vi "函数类型3测试.vi"() -> ()   [LabVIEW 2010]
uses:
  全局量/试验配置信息.vi
panel:
  out "合格？":bool[](array[boolean])
  in  "第几组数据":i32
  out "D_IN_1 2":string[][](table) caption="表格"
  in  "加载文件名称":string
  out "配置文件路径":path
  out "配置文件目录 2":path
  out "配置文件目录":path
  in  "加载配置文件":u16(ring)
  in  "同步_A2":i32
  in  "同步_A1":i32
  in  "数组_输入值":enum16{"0", "1"}[](array[ring])
  in  "数组_选择?":bool[](array[boolean])
  in  "btn_置1_5":bool
  in  "btn_置1_4":bool
  in  "btn_置1_3":bool
  in  "btn_置1_2":bool
  in  "btn_全选_5":bool
  in  "btn_全选_4":bool
  in  "btn_全选_3":bool
  in  "btn_全选_2":bool
  in  "btn_置1_1":bool
  in  "btn_全选_1":bool
  in  "CAN端口":u16
  out "light_80":bool
  out "light_79":bool
  out "light_78":bool
  out "light_77":bool
  out "light_76":bool
  out "light_75":bool
  out "light_74":bool
  out "light_73":bool
  out "light_72":bool
  out "light_71":bool
  out "light_70":bool
  out "light_69":bool
  out "light_68":bool
  out "light_67":bool
  out "light_66":bool
  out "light_65":bool
  in  "输入值_73":enum16{"0", "1"}(ring)
  in  "输入值_80":enum16{"0", "1"}(ring)
  in  "输入值_79":enum16{"0", "1"}(ring)
  in  "输入值_78":enum16{"0", "1"}(ring)
  in  "输入值_77":enum16{"0", "1"}(ring)
  in  "输入值_76":enum16{"0", "1"}(ring)
  in  "输入值_75":enum16{"0", "1"}(ring)
  in  "输入值_74":enum16{"0", "1"}(ring)
  in  "输入值_65":enum16{"0", "1"}(ring)
  in  "输入值_72":enum16{"0", "1"}(ring)
  in  "输入值_71":enum16{"0", "1"}(ring)
  in  "输入值_70":enum16{"0", "1"}(ring)
  in  "输入值_69":enum16{"0", "1"}(ring)
  in  "输入值_68":enum16{"0", "1"}(ring)
  in  "输入值_67":enum16{"0", "1"}(ring)
  in  "输入值_66":enum16{"0", "1"}(ring)
  in  "单选_第73路":bool
  in  "单选_第80路":bool
  in  "单选_第79路":bool
  in  "单选_第78路":bool
  in  "单选_第77路":bool
  in  "单选_第76路":bool
  in  "单选_第75路":bool
  in  "单选_第74路":bool
  in  "单选_第65路":bool
  in  "单选_第72路":bool
  in  "单选_第71路":bool
  in  "单选_第70路":bool
  in  "单选_第69路":bool
  in  "单选_第68路":bool
  in  "单选_第67路":bool
  in  "单选_第66路":bool
  out "light_64":bool
  out "light_63":bool
  out "light_62":bool
  out "light_61":bool
  out "light_60":bool
  out "light_59":bool
  out "light_58":bool
  out "light_57":bool
  out "light_56":bool
  out "light_55":bool
  out "light_54":bool
  out "light_53":bool
  out "light_52":bool
  out "light_51":bool
  out "light_50":bool
  out "light_49":bool
  in  "输入值_57":enum16{"0", "1"}(ring)
  in  "输入值_64":enum16{"0", "1"}(ring)
  in  "输入值_63":enum16{"0", "1"}(ring)
  in  "输入值_62":enum16{"0", "1"}(ring)
  in  "输入值_61":enum16{"0", "1"}(ring)
  in  "输入值_60":enum16{"0", "1"}(ring)
  in  "输入值_59":enum16{"0", "1"}(ring)
  in  "输入值_58":enum16{"0", "1"}(ring)
  in  "输入值_49":enum16{"0", "1"}(ring)
  in  "输入值_56":enum16{"0", "1"}(ring)
  in  "输入值_55":enum16{"0", "1"}(ring)
  in  "输入值_54":enum16{"0", "1"}(ring)
  in  "输入值_53":enum16{"0", "1"}(ring)
  in  "输入值_52":enum16{"0", "1"}(ring)
  in  "输入值_51":enum16{"0", "1"}(ring)
  in  "输入值_50":enum16{"0", "1"}(ring)
  in  "单选_第57路":bool
  in  "单选_第64路":bool
  in  "单选_第63路":bool
  in  "单选_第62路":bool
  in  "单选_第61路":bool
  in  "单选_第60路":bool
  in  "单选_第59路":bool
  in  "单选_第58路":bool
  in  "单选_第49路":bool
  in  "单选_第56路":bool
  in  "单选_第55路":bool
  in  "单选_第54路":bool
  in  "单选_第53路":bool
  in  "单选_第52路":bool
  in  "单选_第51路":bool
  in  "单选_第50路":bool
  out "light_48":bool
  out "light_47":bool
  out "light_46":bool
  out "light_45":bool
  out "light_44":bool
  out "light_43":bool
  out "light_42":bool
  out "light_41":bool
  out "light_40":bool
  out "light_39":bool
  out "light_38":bool
  out "light_37":bool
  out "light_36":bool
  out "light_35":bool
  out "light_34":bool
  out "light_33":bool
  in  "输入值_41":enum16{"0", "1"}(ring)
  in  "输入值_48":enum16{"0", "1"}(ring)
  in  "输入值_47":enum16{"0", "1"}(ring)
  in  "输入值_46":enum16{"0", "1"}(ring)
  in  "输入值_45":enum16{"0", "1"}(ring)
  in  "输入值_44":enum16{"0", "1"}(ring)
  in  "输入值_43":enum16{"0", "1"}(ring)
  in  "输入值_42":enum16{"0", "1"}(ring)
  in  "输入值_33":enum16{"0", "1"}(ring)
  in  "输入值_40":enum16{"0", "1"}(ring)
  in  "输入值_39":enum16{"0", "1"}(ring)
  in  "输入值_38":enum16{"0", "1"}(ring)
  in  "输入值_37":enum16{"0", "1"}(ring)
  in  "输入值_36":enum16{"0", "1"}(ring)
  in  "输入值_35":enum16{"0", "1"}(ring)
  in  "输入值_34":enum16{"0", "1"}(ring)
  in  "单选_第41路":bool
  in  "单选_第48路":bool
  in  "单选_第47路":bool
  in  "单选_第46路":bool
  in  "单选_第45路":bool
  in  "单选_第44路":bool
  in  "单选_第43路":bool
  in  "单选_第42路":bool
  in  "单选_第33路":bool
  in  "单选_第40路":bool
  in  "单选_第39路":bool
  in  "单选_第38路":bool
  in  "单选_第37路":bool
  in  "单选_第36路":bool
  in  "单选_第35路":bool
  in  "单选_第34路":bool
  out "light_32":bool
  out "light_31":bool
  out "light_30":bool
  out "light_29":bool
  out "light_28":bool
  out "light_27":bool
  out "light_26":bool
  out "light_25":bool
  out "light_24":bool
  out "light_23":bool
  out "light_22":bool
  out "light_21":bool
  out "light_20":bool
  out "light_19":bool
  out "light_18":bool
  out "light_17":bool
  in  "输入值_25":enum16{"0", "1"}(ring)
  in  "输入值_32":enum16{"0", "1"}(ring)
  in  "输入值_31":enum16{"0", "1"}(ring)
  in  "输入值_30":enum16{"0", "1"}(ring)
  in  "输入值_29":enum16{"0", "1"}(ring)
  in  "输入值_28":enum16{"0", "1"}(ring)
  in  "输入值_27":enum16{"0", "1"}(ring)
  in  "输入值_26":enum16{"0", "1"}(ring)
  in  "输入值_17":enum16{"0", "1"}(ring)
  in  "输入值_24":enum16{"0", "1"}(ring)
  in  "输入值_23":enum16{"0", "1"}(ring)
  in  "输入值_22":enum16{"0", "1"}(ring)
  in  "输入值_21":enum16{"0", "1"}(ring)
  in  "输入值_20":enum16{"0", "1"}(ring)
  in  "输入值_19":enum16{"0", "1"}(ring)
  in  "输入值_18":enum16{"0", "1"}(ring)
  in  "单选_第25路":bool
  in  "单选_第32路":bool
  in  "单选_第31路":bool
  in  "单选_第30路":bool
  in  "单选_第29路":bool
  in  "单选_第28路":bool
  in  "单选_第27路":bool
  in  "单选_第26路":bool
  in  "单选_第17路":bool
  in  "单选_第24路":bool
  in  "单选_第23路":bool
  in  "单选_第22路":bool
  in  "单选_第21路":bool
  in  "单选_第20路":bool
  in  "单选_第19路":bool
  in  "单选_第18路":bool
  in  "D_IN_5":string[][](table) caption="表格"
  in  "D_IN_4":string[][](table) caption="表格"
  in  "D_IN_3":string[][](table) caption="表格"
  in  "D_IN_2":string[][](table) caption="表格"
  out "light_16":bool
  out "light_15":bool
  out "light_14":bool
  out "light_13":bool
  out "light_12":bool
  out "light_11":bool
  out "light_10":bool
  out "light_9":bool
  out "light_8":bool
  out "light_7":bool
  out "light_6":bool
  out "light_5":bool
  out "light_4":bool
  out "light_3":bool
  out "light_2":bool
  out "light_1":bool
  in  "输入值_9":enum16{"0", "1"}(ring)
  in  "输入值_16":enum16{"0", "1"}(ring)
  in  "输入值_15":enum16{"0", "1"}(ring)
  in  "输入值_14":enum16{"0", "1"}(ring)
  in  "输入值_13":enum16{"0", "1"}(ring)
  in  "输入值_12":enum16{"0", "1"}(ring)
  in  "输入值_11":enum16{"0", "1"}(ring)
  in  "输入值_10":enum16{"0", "1"}(ring)
  in  "输入值_1":enum16{"0", "1"}(ring)
  in  "输入值_8":enum16{"0", "1"}(ring)
  in  "输入值_7":enum16{"0", "1"}(ring)
  in  "输入值_6":enum16{"0", "1"}(ring)
  in  "输入值_5":enum16{"0", "1"}(ring)
  in  "输入值_4":enum16{"0", "1"}(ring)
  in  "输入值_3":enum16{"0", "1"}(ring)
  in  "输入值_2":enum16{"0", "1"}(ring)
  in  "单选_第9路":bool
  in  "单选_第16路":bool
  in  "单选_第15路":bool
  in  "单选_第14路":bool
  in  "单选_第13路":bool
  in  "单选_第12路":bool
  in  "单选_第11路":bool
  in  "单选_第10路":bool
  in  "单选_第1路":bool
  in  "单选_第8路":bool
  in  "单选_第7路":bool
  in  "单选_第6路":bool
  in  "单选_第5路":bool
  in  "单选_第4路":bool
  in  "单选_第3路":bool
  in  "单选_第2路":bool
  in  "D_IN_1":string[][](table) caption="表格"
  out "关闭？":bool
  out "测试结论":string
  in  "btn_置0":bool
  in  "btn_置1":bool
  in  "btn_反选":bool
  in  "btn_全选":bool
  in  "btn_关闭":bool
  in  "btn_开始试验":bool
  # "第一组数字量测试"
  # "第二组数字量测试"
  # "第三组数字量测试"
  # "第四组数字量测试"
  # "第五组数字量测试"
  # "加载配置文件："
  # "测试结论："
  # "80"
  # "80"
  # "80"
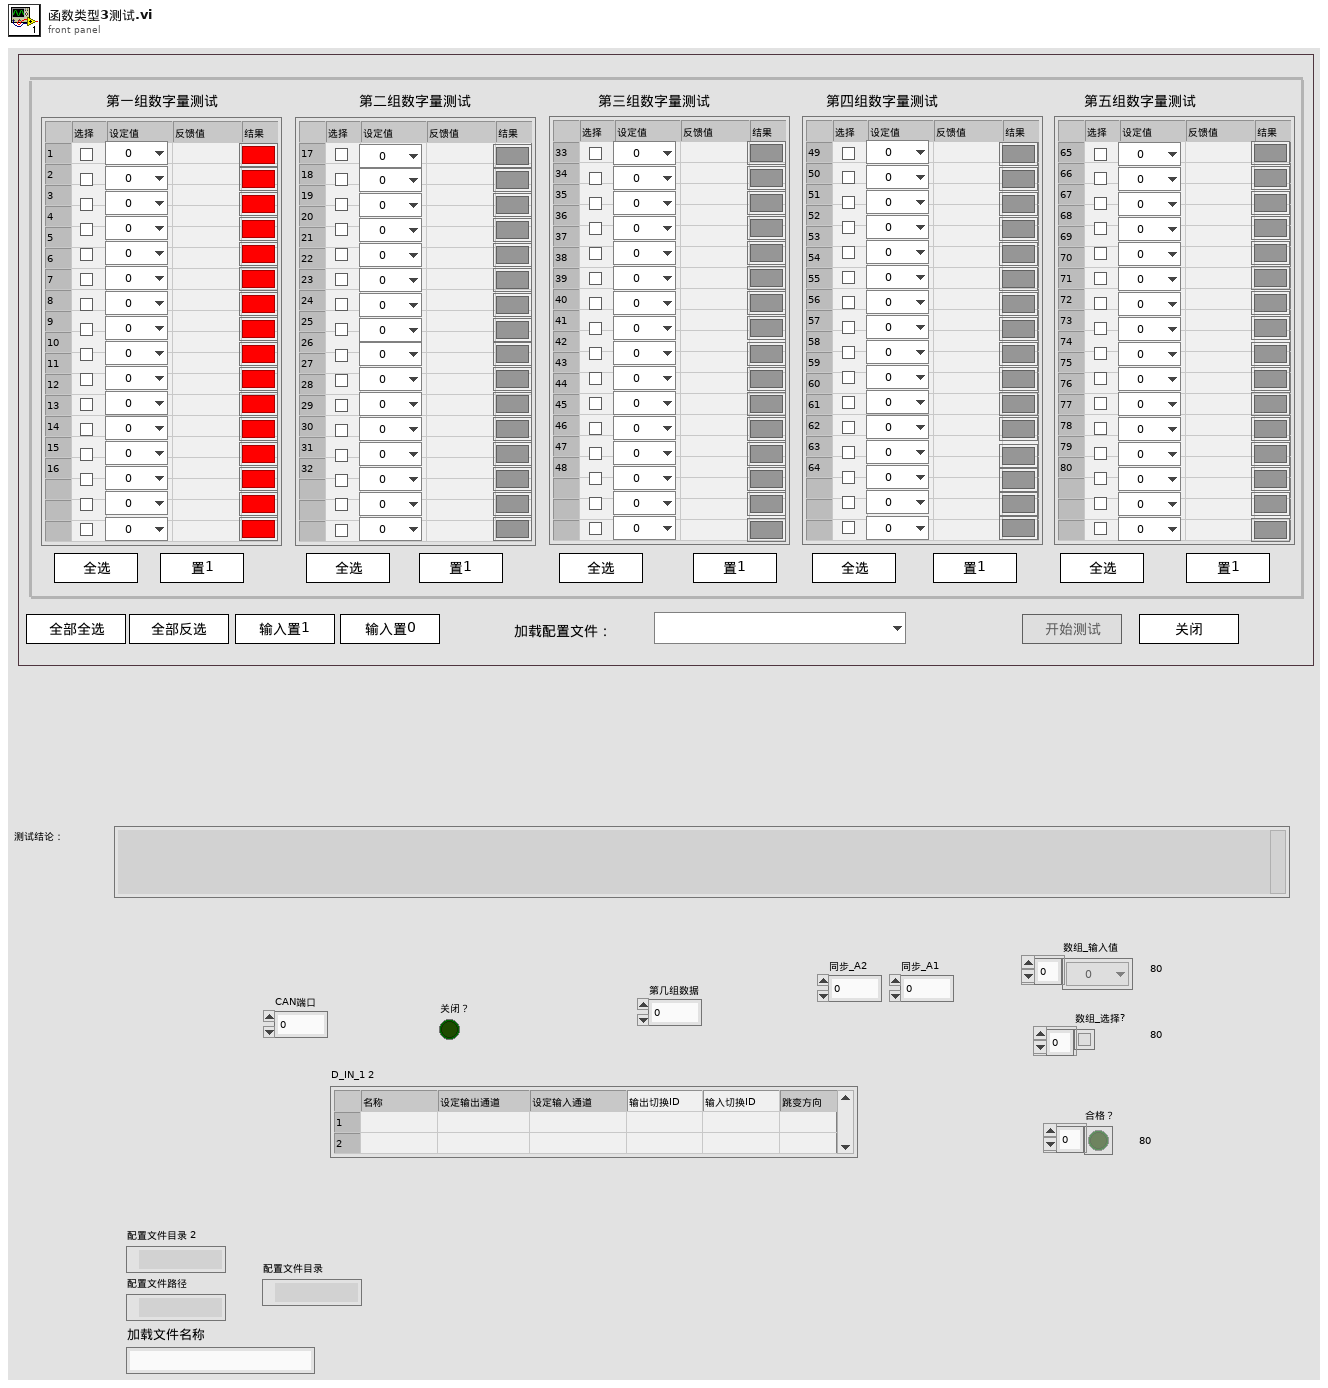
[diagram p1: front panel]
types:
  T1 = enum8{"Enabled", "Disabled", "Disabled and Grayed Out"}
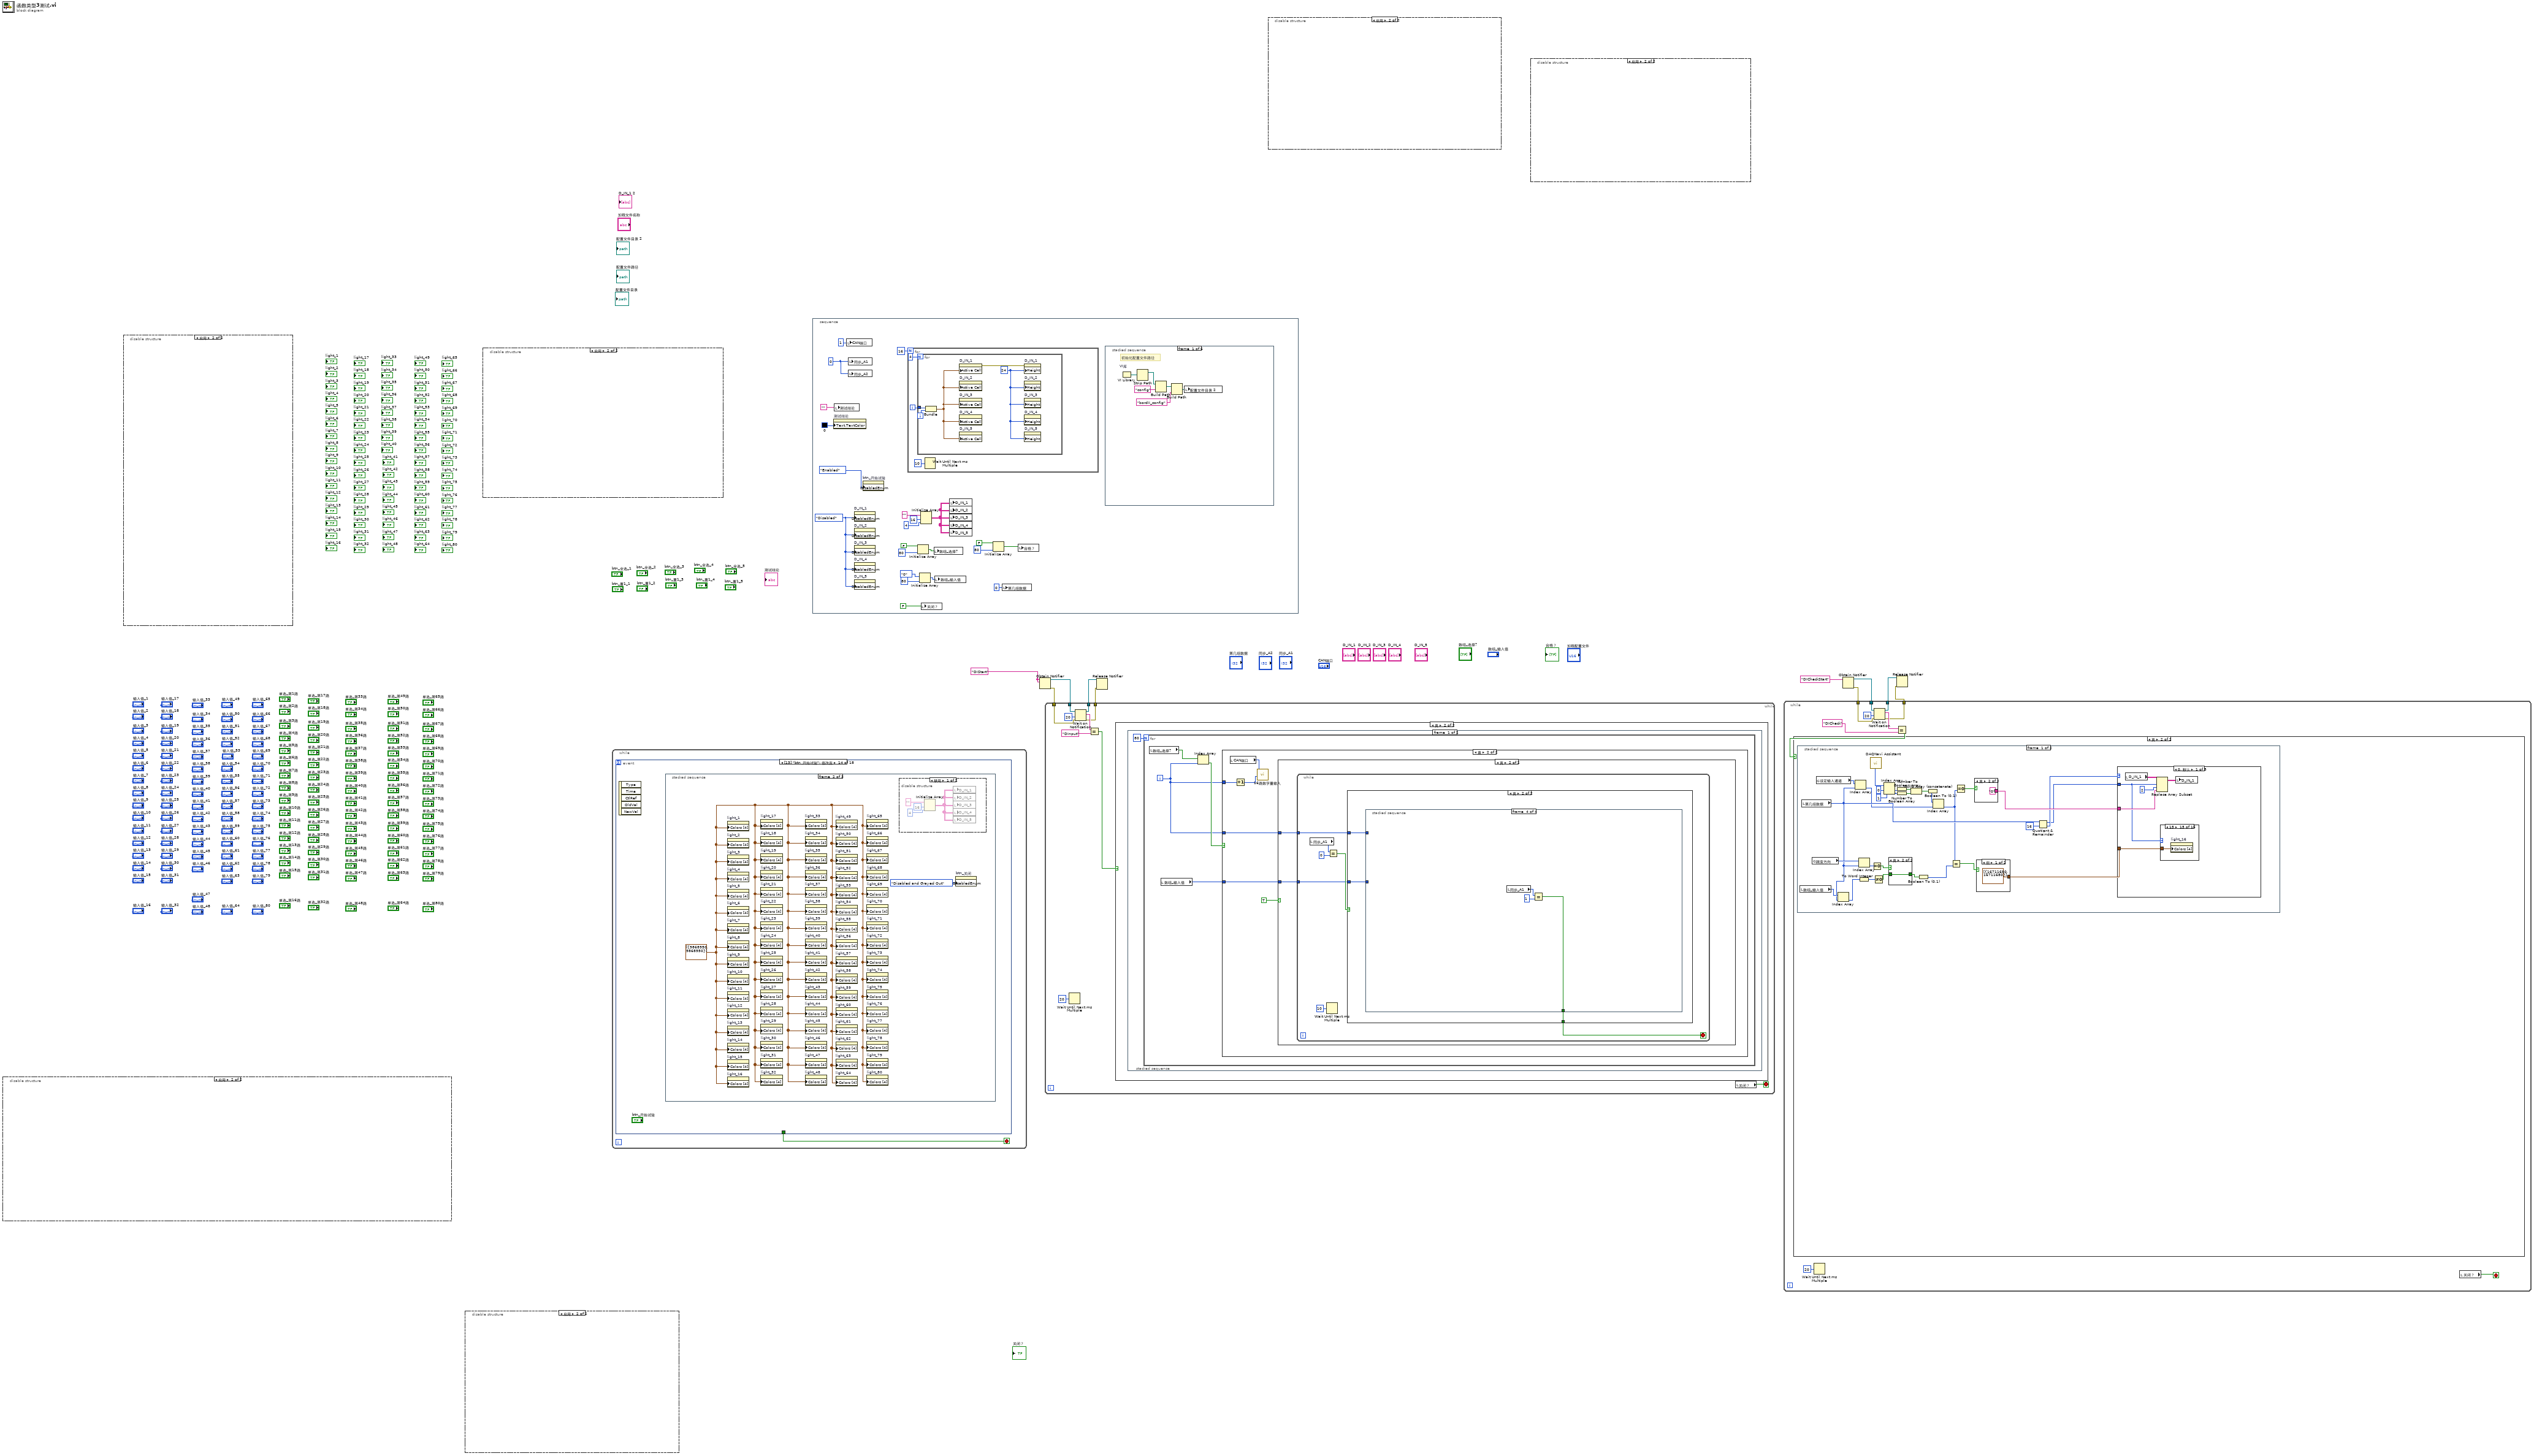
[diagram p0: block diagram]
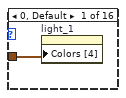
[diagram p3: hidden frame]
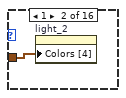
[diagram p4: hidden frame]
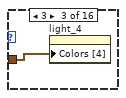
[diagram p5: hidden frame]
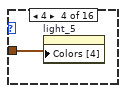
[diagram p6: hidden frame]
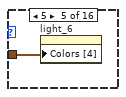
[diagram p7: hidden frame]
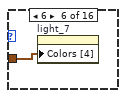
[diagram p8: hidden frame]
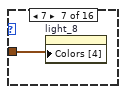
[diagram p9: hidden frame]
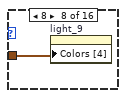
[diagram p10: hidden frame]
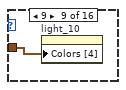
[diagram p11: hidden frame]
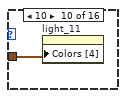
[diagram p12: hidden frame]
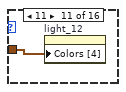
[diagram p13: hidden frame]
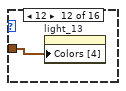
[diagram p14: hidden frame]
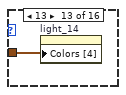
[diagram p15: hidden frame]
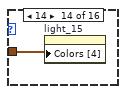
[diagram p16: hidden frame]
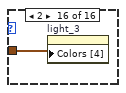
[diagram p17: hidden frame]
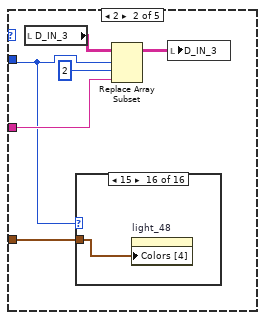
[diagram p18: hidden frame]
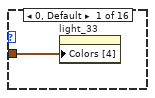
[diagram p19: hidden frame]
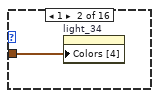
[diagram p20: hidden frame]
diagram:
  w1 = "DICheckStart" ("名称（未命名）")
  w2 = "DIStart" ("名称（未命名）")
  n1 = disable-structure shown="启用" {
    frame Disabled {
      n2 = local read "单选_第1路"() -> ()  [unwired: 1 in]
      n3 = local read "单选_第2路"() -> ()  [unwired: 1 in]
      n4 = local read "单选_第3路"() -> ()  [unwired: 1 in]
      n5 = local read "单选_第4路"() -> ()  [unwired: 1 in]
      n6 = local read "单选_第5路"() -> ()  [unwired: 1 in]
      n7 = local read "单选_第6路"() -> ()  [unwired: 1 in]
      n8 = local read "单选_第7路"() -> ()  [unwired: 1 in]
      n9 = local read "单选_第8路"() -> ()  [unwired: 1 in]
      n10 = local read "单选_第9路"() -> ()  [unwired: 1 in]
      n11 = local read "单选_第10路"() -> ()  [unwired: 1 in]
      n12 = local read "单选_第11路"() -> ()  [unwired: 1 in]
      n13 = local read "单选_第12路"() -> ()  [unwired: 1 in]
      n14 = local read "单选_第13路"() -> ()  [unwired: 1 in]
      n15 = local read "单选_第14路"() -> ()  [unwired: 1 in]
      n16 = local read "单选_第15路"() -> ()  [unwired: 1 in]
      n17 = local read "单选_第16路"() -> ()  [unwired: 1 in]
      n18 = local read "单选_第17路"() -> ()  [unwired: 1 in]
      n19 = local read "单选_第18路"() -> ()  [unwired: 1 in]
      n20 = local read "单选_第19路"() -> ()  [unwired: 1 in]
      n21 = local read "单选_第20路"() -> ()  [unwired: 1 in]
      n22 = local read "单选_第21路"() -> ()  [unwired: 1 in]
      n23 = local read "单选_第22路"() -> ()  [unwired: 1 in]
      n24 = local read "单选_第23路"() -> ()  [unwired: 1 in]
      n25 = local read "单选_第24路"() -> ()  [unwired: 1 in]
      n26 = local read "单选_第25路"() -> ()  [unwired: 1 in]
      n27 = local read "单选_第26路"() -> ()  [unwired: 1 in]
      n28 = local read "单选_第27路"() -> ()  [unwired: 1 in]
      n29 = local read "单选_第28路"() -> ()  [unwired: 1 in]
      n30 = local read "单选_第29路"() -> ()  [unwired: 1 in]
      n31 = local read "单选_第30路"() -> ()  [unwired: 1 in]
      n32 = local read "单选_第31路"() -> ()  [unwired: 1 in]
      n33 = local read "单选_第32路"() -> ()  [unwired: 1 in]
      n34 = local read "单选_第33路"() -> ()  [unwired: 1 in]
      n35 = local read "单选_第34路"() -> ()  [unwired: 1 in]
      n36 = local read "单选_第35路"() -> ()  [unwired: 1 in]
      n37 = local read "单选_第36路"() -> ()  [unwired: 1 in]
      n38 = local read "单选_第37路"() -> ()  [unwired: 1 in]
      n39 = local read "单选_第38路"() -> ()  [unwired: 1 in]
      n40 = local read "单选_第39路"() -> ()  [unwired: 1 in]
      n41 = local read "单选_第40路"() -> ()  [unwired: 1 in]
      n42 = local read "单选_第41路"() -> ()  [unwired: 1 in]
      n43 = local read "单选_第42路"() -> ()  [unwired: 1 in]
      n44 = local read "单选_第43路"() -> ()  [unwired: 1 in]
      n45 = local read "单选_第44路"() -> ()  [unwired: 1 in]
      n46 = local read "单选_第45路"() -> ()  [unwired: 1 in]
      n47 = local read "单选_第46路"() -> ()  [unwired: 1 in]
      n48 = local read "单选_第47路"() -> ()  [unwired: 1 in]
      n49 = local read "单选_第48路"() -> ()  [unwired: 1 in]
      n50 = local read "单选_第49路"() -> ()  [unwired: 1 in]
      n51 = local read "单选_第50路"() -> ()  [unwired: 1 in]
      n52 = local read "单选_第51路"() -> ()  [unwired: 1 in]
      n53 = local read "单选_第52路"() -> ()  [unwired: 1 in]
      n54 = local read "单选_第53路"() -> ()  [unwired: 1 in]
      n55 = local read "单选_第54路"() -> ()  [unwired: 1 in]
      n56 = local read "单选_第55路"() -> ()  [unwired: 1 in]
      n57 = local read "单选_第56路"() -> ()  [unwired: 1 in]
      n58 = local read "单选_第57路"() -> ()  [unwired: 1 in]
      n59 = local read "单选_第58路"() -> ()  [unwired: 1 in]
      n60 = local read "单选_第59路"() -> ()  [unwired: 1 in]
      n61 = local read "单选_第60路"() -> ()  [unwired: 1 in]
      n62 = local read "单选_第61路"() -> ()  [unwired: 1 in]
      n63 = local read "单选_第62路"() -> ()  [unwired: 1 in]
      n64 = local read "单选_第63路"() -> ()  [unwired: 1 in]
      n65 = local read "单选_第64路"() -> ()  [unwired: 1 in]
      n66 = local read "单选_第71路"() -> ()  [unwired: 1 in]
      n67 = local read "单选_第79路"() -> ()  [unwired: 1 in]
      n68 = local read "单选_第65路"() -> ()  [unwired: 1 in]
      n69 = local read "单选_第66路"() -> ()  [unwired: 1 in]
      n70 = local read "单选_第67路"() -> ()  [unwired: 1 in]
      n71 = local read "单选_第68路"() -> ()  [unwired: 1 in]
      n72 = local read "单选_第69路"() -> ()  [unwired: 1 in]
      n73 = local read "单选_第70路"() -> ()  [unwired: 1 in]
      n74 = local read "单选_第72路"() -> ()  [unwired: 1 in]
      n75 = local read "单选_第73路"() -> ()  [unwired: 1 in]
      n76 = local read "单选_第74路"() -> ()  [unwired: 1 in]
      n77 = local read "单选_第75路"() -> ()  [unwired: 1 in]
      n78 = local read "单选_第76路"() -> ()  [unwired: 1 in]
      n79 = local read "单选_第77路"() -> ()  [unwired: 1 in]
      n80 = local read "单选_第78路"() -> ()  [unwired: 1 in]
      n81 = local read "单选_第80路"() -> ()  [unwired: 1 in]
      n82 = local read "输入值_1"() -> ()  [unwired: 1 in]
      n83 = local read "输入值_2"() -> ()  [unwired: 1 in]
      n84 = local read "输入值_3"() -> ()  [unwired: 1 in]
      n85 = local read "输入值_4"() -> ()  [unwired: 1 in]
      n86 = local read "输入值_5"() -> ()  [unwired: 1 in]
      n87 = local read "输入值_6"() -> ()  [unwired: 1 in]
      n88 = local read "输入值_7"() -> ()  [unwired: 1 in]
      n89 = local read "输入值_8"() -> ()  [unwired: 1 in]
      n90 = local read "输入值_9"() -> ()  [unwired: 1 in]
      n91 = local read "输入值_10"() -> ()  [unwired: 1 in]
      n92 = local read "输入值_11"() -> ()  [unwired: 1 in]
      n93 = local read "输入值_12"() -> ()  [unwired: 1 in]
      n94 = local read "输入值_13"() -> ()  [unwired: 1 in]
      n95 = local read "输入值_14"() -> ()  [unwired: 1 in]
      n96 = local read "输入值_15"() -> ()  [unwired: 1 in]
      n97 = local read "输入值_16"() -> ()  [unwired: 1 in]
      n98 = local read "输入值_17"() -> ()  [unwired: 1 in]
      n99 = local read "输入值_18"() -> ()  [unwired: 1 in]
      n100 = local read "输入值_19"() -> ()  [unwired: 1 in]
      n101 = local read "输入值_20"() -> ()  [unwired: 1 in]
      n102 = local read "输入值_21"() -> ()  [unwired: 1 in]
      n103 = local read "输入值_22"() -> ()  [unwired: 1 in]
      n104 = local read "输入值_23"() -> ()  [unwired: 1 in]
      n105 = local read "输入值_24"() -> ()  [unwired: 1 in]
      n106 = local read "输入值_25"() -> ()  [unwired: 1 in]
      n107 = local read "输入值_26"() -> ()  [unwired: 1 in]
      n108 = local read "输入值_27"() -> ()  [unwired: 1 in]
      n109 = local read "输入值_28"() -> ()  [unwired: 1 in]
      n110 = local read "输入值_29"() -> ()  [unwired: 1 in]
      n111 = local read "输入值_30"() -> ()  [unwired: 1 in]
      n112 = local read "输入值_31"() -> ()  [unwired: 1 in]
      n113 = local read "输入值_32"() -> ()  [unwired: 1 in]
      n114 = local read "输入值_33"() -> ()  [unwired: 1 in]
      n115 = local read "输入值_34"() -> ()  [unwired: 1 in]
      n116 = local read "输入值_35"() -> ()  [unwired: 1 in]
      n117 = local read "输入值_36"() -> ()  [unwired: 1 in]
      n118 = local read "输入值_37"() -> ()  [unwired: 1 in]
      n119 = local read "输入值_38"() -> ()  [unwired: 1 in]
      n120 = local read "输入值_39"() -> ()  [unwired: 1 in]
      n121 = local read "输入值_40"() -> ()  [unwired: 1 in]
      n122 = local read "输入值_41"() -> ()  [unwired: 1 in]
      n123 = local read "输入值_42"() -> ()  [unwired: 1 in]
      n124 = local read "输入值_43"() -> ()  [unwired: 1 in]
      n125 = local read "输入值_44"() -> ()  [unwired: 1 in]
      n126 = local read "输入值_45"() -> ()  [unwired: 1 in]
      n127 = local read "输入值_46"() -> ()  [unwired: 1 in]
      n128 = local read "输入值_47"() -> ()  [unwired: 1 in]
      n129 = local read "输入值_48"() -> ()  [unwired: 1 in]
      n130 = local read "输入值_49"() -> ()  [unwired: 1 in]
      n131 = local read "输入值_50"() -> ()  [unwired: 1 in]
      n132 = local read "输入值_51"() -> ()  [unwired: 1 in]
      n133 = local read "输入值_52"() -> ()  [unwired: 1 in]
      n134 = local read "输入值_53"() -> ()  [unwired: 1 in]
      n135 = local read "输入值_54"() -> ()  [unwired: 1 in]
      n136 = local read "输入值_55"() -> ()  [unwired: 1 in]
      n137 = local read "输入值_56"() -> ()  [unwired: 1 in]
      n138 = local read "输入值_57"() -> ()  [unwired: 1 in]
      n139 = local read "输入值_58"() -> ()  [unwired: 1 in]
      n140 = local read "输入值_59"() -> ()  [unwired: 1 in]
      n141 = local read "输入值_60"() -> ()  [unwired: 1 in]
      n142 = local read "输入值_61"() -> ()  [unwired: 1 in]
      n143 = local read "输入值_62"() -> ()  [unwired: 1 in]
      n144 = local read "输入值_63"() -> ()  [unwired: 1 in]
      n145 = local read "输入值_64"() -> ()  [unwired: 1 in]
      n146 = local read "输入值_65"() -> ()  [unwired: 1 in]
      n147 = local read "输入值_66"() -> ()  [unwired: 1 in]
      n148 = local read "输入值_67"() -> ()  [unwired: 1 in]
      n149 = local read "输入值_68"() -> ()  [unwired: 1 in]
      n150 = local read "输入值_69"() -> ()  [unwired: 1 in]
      n151 = local read "输入值_70"() -> ()  [unwired: 1 in]
      n152 = local read "输入值_71"() -> ()  [unwired: 1 in]
      n153 = local read "输入值_72"() -> ()  [unwired: 1 in]
      n154 = local read "输入值_73"() -> ()  [unwired: 1 in]
      n155 = local read "输入值_74"() -> ()  [unwired: 1 in]
      n156 = local read "输入值_75"() -> ()  [unwired: 1 in]
      n157 = local read "输入值_76"() -> ()  [unwired: 1 in]
      n158 = local read "输入值_77"() -> ()  [unwired: 1 in]
      n159 = local read "输入值_78"() -> ()  [unwired: 1 in]
      n160 = local read "输入值_79"() -> ()  [unwired: 1 in]
      n161 = local read "输入值_80"() -> ()  [unwired: 1 in]
    }
    frame Enabled {
    }
  }
  n162 = disable-structure shown="启用" {
    frame Disabled {
      n163 = property on="light_1" class="Bool (严格)" props=["Colors [4]"]() -> ()  [unwired: 3 in, 2 out]
      n164 = property on="light_2" class="Bool (严格)" props=["Colors [4]"]() -> ()  [unwired: 3 in, 2 out]
      n165 = property on="light_3" class="Bool (严格)" props=["Colors [4]"]() -> ()  [unwired: 3 in, 2 out]
      n166 = property on="light_4" class="Bool (严格)" props=["Colors [4]"]() -> ()  [unwired: 3 in, 2 out]
      n167 = property on="light_5" class="Bool (严格)" props=["Colors [4]"]() -> ()  [unwired: 3 in, 2 out]
      n168 = property on="light_6" class="Bool (严格)" props=["Colors [4]"]() -> ()  [unwired: 3 in, 2 out]
      n169 = property on="light_7" class="Bool (严格)" props=["Colors [4]"]() -> ()  [unwired: 3 in, 2 out]
      n170 = property on="light_8" class="Bool (严格)" props=["Colors [4]"]() -> ()  [unwired: 3 in, 2 out]
      n171 = property on="light_9" class="Bool (严格)" props=["Colors [4]"]() -> ()  [unwired: 3 in, 2 out]
      n172 = property on="light_10" class="Bool (严格)" props=["Colors [4]"]() -> ()  [unwired: 3 in, 2 out]
      n173 = property on="light_11" class="Bool (严格)" props=["Colors [4]"]() -> ()  [unwired: 3 in, 2 out]
      n174 = property on="light_12" class="Bool (严格)" props=["Colors [4]"]() -> ()  [unwired: 3 in, 2 out]
      n175 = property on="light_13" class="Bool (严格)" props=["Colors [4]"]() -> ()  [unwired: 3 in, 2 out]
      n176 = property on="light_14" class="Bool (严格)" props=["Colors [4]"]() -> ()  [unwired: 3 in, 2 out]
      n177 = property on="light_15" class="Bool (严格)" props=["Colors [4]"]() -> ()  [unwired: 3 in, 2 out]
      n178 = property on="light_16" class="Bool (严格)" props=["Colors [4]"]() -> ()  [unwired: 3 in, 2 out]
      n179 = property on="light_17" class="Bool (严格)" props=["Colors [4]"]() -> ()  [unwired: 3 in, 2 out]
      n180 = property on="light_18" class="Bool (严格)" props=["Colors [4]"]() -> ()  [unwired: 3 in, 2 out]
      n181 = property on="light_19" class="Bool (严格)" props=["Colors [4]"]() -> ()  [unwired: 3 in, 2 out]
      n182 = property on="light_20" class="Bool (严格)" props=["Colors [4]"]() -> ()  [unwired: 3 in, 2 out]
      n183 = property on="light_21" class="Bool (严格)" props=["Colors [4]"]() -> ()  [unwired: 3 in, 2 out]
      n184 = property on="light_22" class="Bool (严格)" props=["Colors [4]"]() -> ()  [unwired: 3 in, 2 out]
      n185 = property on="light_23" class="Bool (严格)" props=["Colors [4]"]() -> ()  [unwired: 3 in, 2 out]
      n186 = property on="light_24" class="Bool (严格)" props=["Colors [4]"]() -> ()  [unwired: 3 in, 2 out]
      n187 = property on="light_25" class="Bool (严格)" props=["Colors [4]"]() -> ()  [unwired: 3 in, 2 out]
      n188 = property on="light_26" class="Bool (严格)" props=["Colors [4]"]() -> ()  [unwired: 3 in, 2 out]
      n189 = property on="light_27" class="Bool (严格)" props=["Colors [4]"]() -> ()  [unwired: 3 in, 2 out]
      n190 = property on="light_28" class="Bool (严格)" props=["Colors [4]"]() -> ()  [unwired: 3 in, 2 out]
      n191 = property on="light_29" class="Bool (严格)" props=["Colors [4]"]() -> ()  [unwired: 3 in, 2 out]
      n192 = property on="light_30" class="Bool (严格)" props=["Colors [4]"]() -> ()  [unwired: 3 in, 2 out]
      n193 = property on="light_31" class="Bool (严格)" props=["Colors [4]"]() -> ()  [unwired: 3 in, 2 out]
      n194 = property on="light_32" class="Bool (严格)" props=["Colors [4]"]() -> ()  [unwired: 3 in, 2 out]
      n195 = property on="light_33" class="Bool (严格)" props=["Colors [4]"]() -> ()  [unwired: 3 in, 2 out]
      n196 = property on="light_34" class="Bool (严格)" props=["Colors [4]"]() -> ()  [unwired: 3 in, 2 out]
      n197 = property on="light_35" class="Bool (严格)" props=["Colors [4]"]() -> ()  [unwired: 3 in, 2 out]
      n198 = property on="light_36" class="Bool (严格)" props=["Colors [4]"]() -> ()  [unwired: 3 in, 2 out]
      n199 = property on="light_37" class="Bool (严格)" props=["Colors [4]"]() -> ()  [unwired: 3 in, 2 out]
      n200 = property on="light_38" class="Bool (严格)" props=["Colors [4]"]() -> ()  [unwired: 3 in, 2 out]
      n201 = property on="light_39" class="Bool (严格)" props=["Colors [4]"]() -> ()  [unwired: 3 in, 2 out]
      n202 = property on="light_40" class="Bool (严格)" props=["Colors [4]"]() -> ()  [unwired: 3 in, 2 out]
      n203 = property on="light_41" class="Bool (严格)" props=["Colors [4]"]() -> ()  [unwired: 3 in, 2 out]
      n204 = property on="light_42" class="Bool (严格)" props=["Colors [4]"]() -> ()  [unwired: 3 in, 2 out]
      n205 = property on="light_43" class="Bool (严格)" props=["Colors [4]"]() -> ()  [unwired: 3 in, 2 out]
      n206 = property on="light_44" class="Bool (严格)" props=["Colors [4]"]() -> ()  [unwired: 3 in, 2 out]
      n207 = property on="light_45" class="Bool (严格)" props=["Colors [4]"]() -> ()  [unwired: 3 in, 2 out]
      n208 = property on="light_46" class="Bool (严格)" props=["Colors [4]"]() -> ()  [unwired: 3 in, 2 out]
      n209 = property on="light_47" class="Bool (严格)" props=["Colors [4]"]() -> ()  [unwired: 3 in, 2 out]
      n210 = property on="light_48" class="Bool (严格)" props=["Colors [4]"]() -> ()  [unwired: 3 in, 2 out]
      n211 = property on="light_49" class="Bool (严格)" props=["Colors [4]"]() -> ()  [unwired: 3 in, 2 out]
      n212 = property on="light_50" class="Bool (严格)" props=["Colors [4]"]() -> ()  [unwired: 3 in, 2 out]
      n213 = property on="light_51" class="Bool (严格)" props=["Colors [4]"]() -> ()  [unwired: 3 in, 2 out]
      n214 = property on="light_52" class="Bool (严格)" props=["Colors [4]"]() -> ()  [unwired: 3 in, 2 out]
      n215 = property on="light_53" class="Bool (严格)" props=["Colors [4]"]() -> ()  [unwired: 3 in, 2 out]
      n216 = property on="light_54" class="Bool (严格)" props=["Colors [4]"]() -> ()  [unwired: 3 in, 2 out]
      n217 = property on="light_55" class="Bool (严格)" props=["Colors [4]"]() -> ()  [unwired: 3 in, 2 out]
      n218 = property on="light_56" class="Bool (严格)" props=["Colors [4]"]() -> ()  [unwired: 3 in, 2 out]
      n219 = property on="light_57" class="Bool (严格)" props=["Colors [4]"]() -> ()  [unwired: 3 in, 2 out]
      n220 = property on="light_58" class="Bool (严格)" props=["Colors [4]"]() -> ()  [unwired: 3 in, 2 out]
      n221 = property on="light_59" class="Bool (严格)" props=["Colors [4]"]() -> ()  [unwired: 3 in, 2 out]
      n222 = property on="light_60" class="Bool (严格)" props=["Colors [4]"]() -> ()  [unwired: 3 in, 2 out]
      n223 = property on="light_61" class="Bool (严格)" props=["Colors [4]"]() -> ()  [unwired: 3 in, 2 out]
      n224 = property on="light_62" class="Bool (严格)" props=["Colors [4]"]() -> ()  [unwired: 3 in, 2 out]
      n225 = property on="light_63" class="Bool (严格)" props=["Colors [4]"]() -> ()  [unwired: 3 in, 2 out]
      n226 = property on="light_64" class="Bool (严格)" props=["Colors [4]"]() -> ()  [unwired: 3 in, 2 out]
      n227 = property on="light_65" class="Bool (严格)" props=["Colors [4]"]() -> ()  [unwired: 3 in, 2 out]
      n228 = property on="light_66" class="Bool (严格)" props=["Colors [4]"]() -> ()  [unwired: 3 in, 2 out]
      n229 = property on="light_67" class="Bool (严格)" props=["Colors [4]"]() -> ()  [unwired: 3 in, 2 out]
      n230 = property on="light_68" class="Bool (严格)" props=["Colors [4]"]() -> ()  [unwired: 3 in, 2 out]
      n231 = property on="light_69" class="Bool (严格)" props=["Colors [4]"]() -> ()  [unwired: 3 in, 2 out]
      n232 = property on="light_70" class="Bool (严格)" props=["Colors [4]"]() -> ()  [unwired: 3 in, 2 out]
      n233 = property on="light_71" class="Bool (严格)" props=["Colors [4]"]() -> ()  [unwired: 3 in, 2 out]
      n234 = property on="light_72" class="Bool (严格)" props=["Colors [4]"]() -> ()  [unwired: 3 in, 2 out]
      n235 = property on="light_73" class="Bool (严格)" props=["Colors [4]"]() -> ()  [unwired: 3 in, 2 out]
      n236 = property on="light_74" class="Bool (严格)" props=["Colors [4]"]() -> ()  [unwired: 3 in, 2 out]
      n237 = property on="light_75" class="Bool (严格)" props=["Colors [4]"]() -> ()  [unwired: 3 in, 2 out]
      n238 = property on="light_76" class="Bool (严格)" props=["Colors [4]"]() -> ()  [unwired: 3 in, 2 out]
      n239 = property on="light_77" class="Bool (严格)" props=["Colors [4]"]() -> ()  [unwired: 3 in, 2 out]
      n240 = property on="light_78" class="Bool (严格)" props=["Colors [4]"]() -> ()  [unwired: 3 in, 2 out]
      n241 = property on="light_79" class="Bool (严格)" props=["Colors [4]"]() -> ()  [unwired: 3 in, 2 out]
      n242 = property on="light_80" class="Bool (严格)" props=["Colors [4]"]() -> ()  [unwired: 3 in, 2 out]
    }
    frame Enabled {
    }
  }
  n243 = disable-structure shown="启用" {
    frame Disabled {
      n244 = local read "输入值_1"() -> ()  [unwired: 1 out]
      n245 = local read "输入值_2"() -> ()  [unwired: 1 out]
      n246 = local read "输入值_3"() -> ()  [unwired: 1 out]
      n247 = local read "输入值_4"() -> ()  [unwired: 1 out]
      n248 = local read "输入值_5"() -> ()  [unwired: 1 out]
      n249 = local read "输入值_6"() -> ()  [unwired: 1 out]
      n250 = local read "输入值_7"() -> ()  [unwired: 1 out]
      n251 = local read "输入值_8"() -> ()  [unwired: 1 out]
      n252 = local read "输入值_9"() -> ()  [unwired: 1 out]
      n253 = local read "输入值_10"() -> ()  [unwired: 1 out]
      n254 = local read "输入值_11"() -> ()  [unwired: 1 out]
      n255 = local read "输入值_12"() -> ()  [unwired: 1 out]
      n256 = local read "输入值_13"() -> ()  [unwired: 1 out]
      n257 = local read "输入值_14"() -> ()  [unwired: 1 out]
      n258 = local read "输入值_15"() -> ()  [unwired: 1 out]
      n259 = local read "输入值_16"() -> ()  [unwired: 1 out]
      n260 = local read "输入值_17"() -> ()  [unwired: 1 out]
      n261 = local read "输入值_18"() -> ()  [unwired: 1 out]
      n262 = local read "输入值_19"() -> ()  [unwired: 1 out]
      n263 = local read "输入值_20"() -> ()  [unwired: 1 out]
      n264 = local read "输入值_21"() -> ()  [unwired: 1 out]
      n265 = local read "输入值_22"() -> ()  [unwired: 1 out]
      n266 = local read "输入值_23"() -> ()  [unwired: 1 out]
      n267 = local read "输入值_24"() -> ()  [unwired: 1 out]
      n268 = local read "输入值_25"() -> ()  [unwired: 1 out]
      n269 = local read "输入值_26"() -> ()  [unwired: 1 out]
      n270 = local read "输入值_27"() -> ()  [unwired: 1 out]
      n271 = local read "输入值_28"() -> ()  [unwired: 1 out]
      n272 = local read "输入值_29"() -> ()  [unwired: 1 out]
      n273 = local read "输入值_30"() -> ()  [unwired: 1 out]
      n274 = local read "输入值_31"() -> ()  [unwired: 1 out]
      n275 = local read "输入值_32"() -> ()  [unwired: 1 out]
      n276 = local read "输入值_33"() -> ()  [unwired: 1 out]
      n277 = local read "输入值_34"() -> ()  [unwired: 1 out]
      n278 = local read "输入值_35"() -> ()  [unwired: 1 out]
      n279 = local read "输入值_36"() -> ()  [unwired: 1 out]
      n280 = local read "输入值_37"() -> ()  [unwired: 1 out]
      n281 = local read "输入值_38"() -> ()  [unwired: 1 out]
      n282 = local read "输入值_39"() -> ()  [unwired: 1 out]
      n283 = local read "输入值_40"() -> ()  [unwired: 1 out]
      n284 = local read "输入值_41"() -> ()  [unwired: 1 out]
      n285 = local read "输入值_42"() -> ()  [unwired: 1 out]
      n286 = local read "输入值_43"() -> ()  [unwired: 1 out]
      n287 = local read "输入值_44"() -> ()  [unwired: 1 out]
      n288 = local read "输入值_45"() -> ()  [unwired: 1 out]
      n289 = local read "输入值_46"() -> ()  [unwired: 1 out]
      n290 = local read "输入值_47"() -> ()  [unwired: 1 out]
      n291 = local read "输入值_48"() -> ()  [unwired: 1 out]
      n292 = local read "输入值_49"() -> ()  [unwired: 1 out]
      n293 = local read "输入值_50"() -> ()  [unwired: 1 out]
      n294 = local read "输入值_51"() -> ()  [unwired: 1 out]
      n295 = local read "输入值_52"() -> ()  [unwired: 1 out]
      n296 = local read "输入值_53"() -> ()  [unwired: 1 out]
      n297 = local read "输入值_54"() -> ()  [unwired: 1 out]
      n298 = local read "输入值_55"() -> ()  [unwired: 1 out]
      n299 = local read "输入值_56"() -> ()  [unwired: 1 out]
      n300 = local read "输入值_57"() -> ()  [unwired: 1 out]
      n301 = local read "输入值_58"() -> ()  [unwired: 1 out]
      n302 = local read "输入值_59"() -> ()  [unwired: 1 out]
      n303 = local read "输入值_60"() -> ()  [unwired: 1 out]
      n304 = local read "输入值_61"() -> ()  [unwired: 1 out]
      n305 = local read "输入值_62"() -> ()  [unwired: 1 out]
      n306 = local read "输入值_63"() -> ()  [unwired: 1 out]
      n307 = local read "输入值_64"() -> ()  [unwired: 1 out]
      n308 = local read "输入值_65"() -> ()  [unwired: 1 out]
      n309 = local read "输入值_66"() -> ()  [unwired: 1 out]
      n310 = local read "输入值_67"() -> ()  [unwired: 1 out]
      n311 = local read "输入值_68"() -> ()  [unwired: 1 out]
      n312 = local read "输入值_69"() -> ()  [unwired: 1 out]
      n313 = local read "输入值_70"() -> ()  [unwired: 1 out]
      n314 = local read "输入值_71"() -> ()  [unwired: 1 out]
      n315 = local read "输入值_72"() -> ()  [unwired: 1 out]
      n316 = local read "输入值_73"() -> ()  [unwired: 1 out]
      n317 = local read "输入值_74"() -> ()  [unwired: 1 out]
      n318 = local read "输入值_75"() -> ()  [unwired: 1 out]
      n319 = local read "输入值_76"() -> ()  [unwired: 1 out]
      n320 = local read "输入值_77"() -> ()  [unwired: 1 out]
      n321 = local read "输入值_78"() -> ()  [unwired: 1 out]
      n322 = local read "输入值_79"() -> ()  [unwired: 1 out]
      n323 = local read "输入值_80"() -> ()  [unwired: 1 out]
    }
    frame Enabled {
    }
  }
  n324 = disable-structure shown="启用" {
    frame Disabled {
      n325 = local read "light_1"() -> ()  [unwired: 1 in]
      n326 = local read "light_2"() -> ()  [unwired: 1 in]
      n327 = local read "light_3"() -> ()  [unwired: 1 in]
      n328 = local read "light_4"() -> ()  [unwired: 1 in]
      n329 = local read "light_5"() -> ()  [unwired: 1 in]
      n330 = local read "light_6"() -> ()  [unwired: 1 in]
      n331 = local read "light_7"() -> ()  [unwired: 1 in]
      n332 = local read "light_8"() -> ()  [unwired: 1 in]
      n333 = local read "light_9"() -> ()  [unwired: 1 in]
      n334 = local read "light_10"() -> ()  [unwired: 1 in]
      n335 = local read "light_11"() -> ()  [unwired: 1 in]
      n336 = local read "light_12"() -> ()  [unwired: 1 in]
      n337 = local read "light_13"() -> ()  [unwired: 1 in]
      n338 = local read "light_14"() -> ()  [unwired: 1 in]
      n339 = local read "light_15"() -> ()  [unwired: 1 in]
      n340 = local read "light_16"() -> ()  [unwired: 1 in]
      n341 = local read "light_17"() -> ()  [unwired: 1 in]
      n342 = local read "light_18"() -> ()  [unwired: 1 in]
      n343 = local read "light_19"() -> ()  [unwired: 1 in]
      n344 = local read "light_20"() -> ()  [unwired: 1 in]
      n345 = local read "light_21"() -> ()  [unwired: 1 in]
      n346 = local read "light_22"() -> ()  [unwired: 1 in]
      n347 = local read "light_23"() -> ()  [unwired: 1 in]
      n348 = local read "light_24"() -> ()  [unwired: 1 in]
      n349 = local read "light_25"() -> ()  [unwired: 1 in]
      n350 = local read "light_26"() -> ()  [unwired: 1 in]
      n351 = local read "light_27"() -> ()  [unwired: 1 in]
      n352 = local read "light_28"() -> ()  [unwired: 1 in]
      n353 = local read "light_29"() -> ()  [unwired: 1 in]
      n354 = local read "light_30"() -> ()  [unwired: 1 in]
      n355 = local read "light_31"() -> ()  [unwired: 1 in]
      n356 = local read "light_32"() -> ()  [unwired: 1 in]
      n357 = local read "light_33"() -> ()  [unwired: 1 in]
      n358 = local read "light_34"() -> ()  [unwired: 1 in]
      n359 = local read "light_35"() -> ()  [unwired: 1 in]
      n360 = local read "light_36"() -> ()  [unwired: 1 in]
      n361 = local read "light_37"() -> ()  [unwired: 1 in]
      n362 = local read "light_38"() -> ()  [unwired: 1 in]
      n363 = local read "light_39"() -> ()  [unwired: 1 in]
      n364 = local read "light_40"() -> ()  [unwired: 1 in]
      n365 = local read "light_41"() -> ()  [unwired: 1 in]
      n366 = local read "light_42"() -> ()  [unwired: 1 in]
      n367 = local read "light_43"() -> ()  [unwired: 1 in]
      n368 = local read "light_44"() -> ()  [unwired: 1 in]
      n369 = local read "light_45"() -> ()  [unwired: 1 in]
      n370 = local read "light_46"() -> ()  [unwired: 1 in]
      n371 = local read "light_47"() -> ()  [unwired: 1 in]
      n372 = local read "light_48"() -> ()  [unwired: 1 in]
      n373 = local read "light_49"() -> ()  [unwired: 1 in]
      n374 = local read "light_50"() -> ()  [unwired: 1 in]
      n375 = local read "light_51"() -> ()  [unwired: 1 in]
      n376 = local read "light_52"() -> ()  [unwired: 1 in]
      n377 = local read "light_53"() -> ()  [unwired: 1 in]
      n378 = local read "light_54"() -> ()  [unwired: 1 in]
      n379 = local read "light_55"() -> ()  [unwired: 1 in]
      n380 = local read "light_56"() -> ()  [unwired: 1 in]
      n381 = local read "light_57"() -> ()  [unwired: 1 in]
      n382 = local read "light_58"() -> ()  [unwired: 1 in]
      n383 = local read "light_59"() -> ()  [unwired: 1 in]
      n384 = local read "light_60"() -> ()  [unwired: 1 in]
      n385 = local read "light_61"() -> ()  [unwired: 1 in]
      n386 = local read "light_62"() -> ()  [unwired: 1 in]
      n387 = local read "light_63"() -> ()  [unwired: 1 in]
      n388 = local read "light_64"() -> ()  [unwired: 1 in]
      n389 = local read "light_65"() -> ()  [unwired: 1 in]
      n390 = local read "light_66"() -> ()  [unwired: 1 in]
      n391 = local read "light_67"() -> ()  [unwired: 1 in]
      n392 = local read "light_68"() -> ()  [unwired: 1 in]
      n393 = local read "light_69"() -> ()  [unwired: 1 in]
      n394 = local read "light_70"() -> ()  [unwired: 1 in]
      n395 = local read "light_71"() -> ()  [unwired: 1 in]
      n396 = local read "light_72"() -> ()  [unwired: 1 in]
      n397 = local read "light_73"() -> ()  [unwired: 1 in]
      n398 = local read "light_74"() -> ()  [unwired: 1 in]
      n399 = local read "light_75"() -> ()  [unwired: 1 in]
      n400 = local read "light_76"() -> ()  [unwired: 1 in]
      n401 = local read "light_77"() -> ()  [unwired: 1 in]
      n402 = local read "light_78"() -> ()  [unwired: 1 in]
      n403 = local read "light_79"() -> ()  [unwired: 1 in]
      n404 = local read "light_80"() -> ()  [unwired: 1 in]
      n405 = call "DAQNavi Assistant"() -> ()  [unwired: 2 in, 18 out]
    }
    frame Enabled {
    }
  }
  n406 = while {
    stop <- w11 stop-if-true
    n407 = event shown="[13] \"btn_开始试验\": 值改变" {
      selector: _ -> [_ _ _ _ _ _ _ _ _ _ _ _ _ _ _ _ _ _]
      dyn-events: _ -> [_ _ _ _ _ _ _ _ _ _ _ _ _ _ _ _ _ _]
      timeout: _ -> [_ _ _ _ _ _ _ _ _ _ _ _ _ _ _ _ _ _]
      tunnel: [_ w12 w13 _ _ _ _ _ _ _ _ _ _ _ _ _ _ _] -> w11
      event Timeout {
        n408 = event-data() -> ()  [unwired: 1 in, 2 out]
      }
      event Panel Close {
        w12 = TRUE ("关闭？")
        n409 = event-data() -> ()  [unwired: 1 in, 3 out]
        n410 = local write "关闭？"(w12) -> ()
      }
      event "btn_关闭": Value Change {
        w13 = TRUE
        n411 = event-data() -> ()  [unwired: 1 in, 5 out]
        n412 = local write "关闭？"(w13) -> ()
      }
      event "btn_全选_1": Value Change {
        n413 = event-data() -> ("NewVal"=w15:bool)  [unwired: 1 in, 4 out]
        n414 = case shown="假" w15 {
          tunnel: [FALSE ("单选_第41路") TRUE ("单选_第41路")] -> w14
          frame False {
          }
          frame True {
          }
        }
        n415 = local write "单选_第1路"(w14) -> ()
        n416 = local write "单选_第2路"(w14) -> ()
        n417 = local write "单选_第3路"(w14) -> ()
        n418 = local write "单选_第4路"(w14) -> ()
        n419 = local write "单选_第5路"(w14) -> ()
        n420 = local write "单选_第6路"(w14) -> ()
        n421 = local write "单选_第7路"(w14) -> ()
        n422 = local write "单选_第8路"(w14) -> ()
        n423 = local write "单选_第9路"(w14) -> ()
        n424 = local write "单选_第10路"(w14) -> ()
        n425 = local write "单选_第11路"(w14) -> ()
        n426 = local write "单选_第12路"(w14) -> ()
        n427 = local write "单选_第13路"(w14) -> ()
        n428 = local write "单选_第14路"(w14) -> ()
        n429 = local write "单选_第15路"(w14) -> ()
        n430 = local write "单选_第16路"(w14) -> ()
      }
      event "btn_全选_2": Value Change {
        n431 = event-data() -> ("NewVal"=w19:bool)  [unwired: 1 in, 4 out]
        n432 = case shown="假" w19 {
          tunnel: [FALSE ("单选_第41路") TRUE ("单选_第41路")] -> w18
          frame False {
          }
          frame True {
          }
        }
        n433 = local write "单选_第17路"(w18) -> ()
        n434 = local write "单选_第18路"(w18) -> ()
        n435 = local write "单选_第19路"(w18) -> ()
        n436 = local write "单选_第20路"(w18) -> ()
        n437 = local write "单选_第21路"(w18) -> ()
        n438 = local write "单选_第22路"(w18) -> ()
        n439 = local write "单选_第23路"(w18) -> ()
        n440 = local write "单选_第24路"(w18) -> ()
        n441 = local write "单选_第25路"(w18) -> ()
        n442 = local write "单选_第26路"(w18) -> ()
        n443 = local write "单选_第27路"(w18) -> ()
        n444 = local write "单选_第28路"(w18) -> ()
        n445 = local write "单选_第29路"(w18) -> ()
        n446 = local write "单选_第30路"(w18) -> ()
        n447 = local write "单选_第31路"(w18) -> ()
        n448 = local write "单选_第32路"(w18) -> ()
      }
      event "btn_全选_3": Value Change {
        n449 = event-data() -> ("NewVal"=w23:bool)  [unwired: 1 in, 4 out]
        n450 = case shown="假" w23 {
          tunnel: [FALSE ("单选_第41路") TRUE ("单选_第41路")] -> w22
          frame False {
          }
          frame True {
          }
        }
        n451 = local write "单选_第33路"(w22) -> ()
        n452 = local write "单选_第34路"(w22) -> ()
        n453 = local write "单选_第35路"(w22) -> ()
        n454 = local write "单选_第36路"(w22) -> ()
        n455 = local write "单选_第37路"(w22) -> ()
        n456 = local write "单选_第38路"(w22) -> ()
        n457 = local write "单选_第39路"(w22) -> ()
        n458 = local write "单选_第40路"(w22) -> ()
        n459 = local write "单选_第41路"(w22) -> ()
        n460 = local write "单选_第42路"(w22) -> ()
        n461 = local write "单选_第43路"(w22) -> ()
        n462 = local write "单选_第44路"(w22) -> ()
        n463 = local write "单选_第45路"(w22) -> ()
        n464 = local write "单选_第46路"(w22) -> ()
        n465 = local write "单选_第47路"(w22) -> ()
        n466 = local write "单选_第48路"(w22) -> ()
      }
      event "btn_全选_4": Value Change {
        n467 = event-data() -> ("NewVal"=w27:bool)  [unwired: 1 in, 4 out]
        n468 = case shown="假" w27 {
          tunnel: [FALSE ("单选_第41路") TRUE ("单选_第41路")] -> w26
          frame False {
          }
          frame True {
          }
        }
        n469 = local write "单选_第49路"(w26) -> ()
        n470 = local write "单选_第50路"(w26) -> ()
        n471 = local write "单选_第51路"(w26) -> ()
        n472 = local write "单选_第52路"(w26) -> ()
        n473 = local write "单选_第53路"(w26) -> ()
        n474 = local write "单选_第54路"(w26) -> ()
        n475 = local write "单选_第55路"(w26) -> ()
        n476 = local write "单选_第56路"(w26) -> ()
        n477 = local write "单选_第57路"(w26) -> ()
        n478 = local write "单选_第58路"(w26) -> ()
        n479 = local write "单选_第59路"(w26) -> ()
        n480 = local write "单选_第60路"(w26) -> ()
        n481 = local write "单选_第61路"(w26) -> ()
        n482 = local write "单选_第62路"(w26) -> ()
        n483 = local write "单选_第63路"(w26) -> ()
        n484 = local write "单选_第64路"(w26) -> ()
      }
      event "btn_全选_5": Value Change {
        n485 = event-data() -> ("NewVal"=w31:bool)  [unwired: 1 in, 4 out]
        n486 = case shown="假" w31 {
          tunnel: [FALSE ("单选_第41路") TRUE ("单选_第41路")] -> w30
          frame False {
          }
          frame True {
          }
        }
        n487 = local write "单选_第71路"(w30) -> ()
        n488 = local write "单选_第79路"(w30) -> ()
        n489 = local write "单选_第65路"(w30) -> ()
        n490 = local write "单选_第66路"(w30) -> ()
        n491 = local write "单选_第67路"(w30) -> ()
        n492 = local write "单选_第68路"(w30) -> ()
        n493 = local write "单选_第69路"(w30) -> ()
        n494 = local write "单选_第70路"(w30) -> ()
        n495 = local write "单选_第72路"(w30) -> ()
        n496 = local write "单选_第73路"(w30) -> ()
        n497 = local write "单选_第74路"(w30) -> ()
        n498 = local write "单选_第75路"(w30) -> ()
        n499 = local write "单选_第76路"(w30) -> ()
        n500 = local write "单选_第77路"(w30) -> ()
        n501 = local write "单选_第78路"(w30) -> ()
        n502 = local write "单选_第80路"(w30) -> ()
      }
      event "btn_置1_1": Value Change {
        n503 = event-data() -> ("NewVal"=w35:bool)  [unwired: 1 in, 4 out]
        n504 = case shown="假" w35 {
          tunnel: [enum16{"0", "1"}."0" ("输入值_41") enum16{"0", "1"}."1" ("输入值_41")] -> w34
          frame False {
          }
          frame True {
          }
        }
        n505 = local write "输入值_1"(w34) -> ()
        n506 = local write "输入值_2"(w34) -> ()
        n507 = local write "输入值_3"(w34) -> ()
        n508 = local write "输入值_4"(w34) -> ()
        n509 = local write "输入值_5"(w34) -> ()
        n510 = local write "输入值_6"(w34) -> ()
        n511 = local write "输入值_7"(w34) -> ()
        n512 = local write "输入值_8"(w34) -> ()
        n513 = local write "输入值_9"(w34) -> ()
        n514 = local write "输入值_10"(w34) -> ()
        n515 = local write "输入值_11"(w34) -> ()
        n516 = local write "输入值_12"(w34) -> ()
        n517 = local write "输入值_13"(w34) -> ()
        n518 = local write "输入值_14"(w34) -> ()
        n519 = local write "输入值_15"(w34) -> ()
        n520 = local write "输入值_16"(w34) -> ()
      }
      event "btn_置1_2": Value Change {
        n521 = event-data() -> ("NewVal"=w39:bool)  [unwired: 1 in, 4 out]
        n522 = case shown="假" w39 {
          tunnel: [enum16{"0", "1"}."0" ("输入值_41") enum16{"0", "1"}."1" ("输入值_41")] -> w38
          frame False {
          }
          frame True {
          }
        }
        n523 = local write "输入值_17"(w38) -> ()
        n524 = local write "输入值_18"(w38) -> ()
        n525 = local write "输入值_19"(w38) -> ()
        n526 = local write "输入值_20"(w38) -> ()
        n527 = local write "输入值_21"(w38) -> ()
        n528 = local write "输入值_22"(w38) -> ()
        n529 = local write "输入值_23"(w38) -> ()
        n530 = local write "输入值_24"(w38) -> ()
        n531 = local write "输入值_25"(w38) -> ()
        n532 = local write "输入值_26"(w38) -> ()
        n533 = local write "输入值_27"(w38) -> ()
        n534 = local write "输入值_28"(w38) -> ()
        n535 = local write "输入值_29"(w38) -> ()
        n536 = local write "输入值_30"(w38) -> ()
        n537 = local write "输入值_31"(w38) -> ()
        n538 = local write "输入值_32"(w38) -> ()
      }
      event "btn_置1_3": Value Change {
        n539 = event-data() -> ("NewVal"=w43:bool)  [unwired: 1 in, 4 out]
        n540 = case shown="假" w43 {
          tunnel: [enum16{"0", "1"}."0" ("输入值_41") enum16{"0", "1"}."1" ("输入值_41")] -> w42
          frame False {
          }
          frame True {
          }
        }
        n541 = local write "输入值_33"(w42) -> ()
        n542 = local write "输入值_34"(w42) -> ()
        n543 = local write "输入值_35"(w42) -> ()
        n544 = local write "输入值_36"(w42) -> ()
        n545 = local write "输入值_37"(w42) -> ()
        n546 = local write "输入值_38"(w42) -> ()
        n547 = local write "输入值_39"(w42) -> ()
        n548 = local write "输入值_40"(w42) -> ()
        n549 = local write "输入值_41"(w42) -> ()
        n550 = local write "输入值_42"(w42) -> ()
        n551 = local write "输入值_43"(w42) -> ()
        n552 = local write "输入值_44"(w42) -> ()
        n553 = local write "输入值_45"(w42) -> ()
        n554 = local write "输入值_46"(w42) -> ()
        n555 = local write "输入值_47"(w42) -> ()
        n556 = local write "输入值_48"(w42) -> ()
      }
      event "btn_置1_4": Value Change {
        n557 = event-data() -> ("NewVal"=w47:bool)  [unwired: 1 in, 4 out]
        n558 = case shown="假" w47 {
          tunnel: [enum16{"0", "1"}."0" ("输入值_41") enum16{"0", "1"}."1" ("输入值_41")] -> w46
          frame False {
          }
          frame True {
          }
        }
        n559 = local write "输入值_49"(w46) -> ()
        n560 = local write "输入值_50"(w46) -> ()
        n561 = local write "输入值_51"(w46) -> ()
        n562 = local write "输入值_52"(w46) -> ()
        n563 = local write "输入值_53"(w46) -> ()
        n564 = local write "输入值_54"(w46) -> ()
        n565 = local write "输入值_55"(w46) -> ()
        n566 = local write "输入值_56"(w46) -> ()
        n567 = local write "输入值_57"(w46) -> ()
        n568 = local write "输入值_58"(w46) -> ()
        n569 = local write "输入值_59"(w46) -> ()
        n570 = local write "输入值_60"(w46) -> ()
        n571 = local write "输入值_61"(w46) -> ()
        n572 = local write "输入值_62"(w46) -> ()
        n573 = local write "输入值_63"(w46) -> ()
        n574 = local write "输入值_64"(w46) -> ()
      }
      event "btn_置1_5": Value Change {
        n575 = event-data() -> ("NewVal"=w51:bool)  [unwired: 1 in, 4 out]
        n576 = case shown="假" w51 {
          tunnel: [enum16{"0", "1"}."0" ("输入值_41") enum16{"0", "1"}."1" ("输入值_41")] -> w50
          frame False {
          }
          frame True {
          }
        }
        n577 = local write "输入值_65"(w50) -> ()
        n578 = local write "输入值_66"(w50) -> ()
        n579 = local write "输入值_67"(w50) -> ()
        n580 = local write "输入值_68"(w50) -> ()
        n581 = local write "输入值_69"(w50) -> ()
        n582 = local write "输入值_70"(w50) -> ()
        n583 = local write "输入值_71"(w50) -> ()
        n584 = local write "输入值_72"(w50) -> ()
        n585 = local write "输入值_73"(w50) -> ()
        n586 = local write "输入值_74"(w50) -> ()
        n587 = local write "输入值_75"(w50) -> ()
        n588 = local write "输入值_76"(w50) -> ()
        n589 = local write "输入值_77"(w50) -> ()
        n590 = local write "输入值_78"(w50) -> ()
        n591 = local write "输入值_79"(w50) -> ()
        n592 = local write "输入值_80"(w50) -> ()
      }
      event "btn_开始试验": Value Change {
        n593 = event-data() -> ()  [unwired: 1 in, 5 out]
        n594 = stacked-sequence {
          frame #0 {
            w68 = 0 ("同步_A1")
            n595 = stacked-sequence {
              tunnel: [w73 _ _ _ _] -> w65
              tunnel: [w72 _ _ _ _] -> w59
              tunnel: [_ w107 _ _ _] -> w64
              tunnel: [_ w106 _ _ _] -> w58
              tunnel: [_ _ w141 _ _] -> w63
              tunnel: [_ _ w140 _ _] -> w57
              tunnel: [_ _ _ w175 _] -> w62
              tunnel: [_ _ _ w174 _] -> w56
              tunnel: [_ _ _ _ w209] -> w61
              tunnel: [_ _ _ _ w208] -> w55
              frame #0 {
                n596 = local read "单选_第1路"() -> (w90:bool)
                n597 = local read "单选_第2路"() -> (w91:bool)
                n598 = local read "单选_第3路"() -> (w92:bool)
                n599 = local read "单选_第4路"() -> (w93:bool)
                n600 = local read "单选_第5路"() -> (w94:bool)
                n601 = local read "单选_第6路"() -> (w95:bool)
                n602 = local read "单选_第7路"() -> (w96:bool)
                n603 = local read "单选_第8路"() -> (w97:bool)
                n604 = local read "单选_第9路"() -> (w98:bool)
                n605 = local read "单选_第10路"() -> (w99:bool)
                n606 = local read "单选_第11路"() -> (w100:bool)
                n607 = local read "单选_第12路"() -> (w101:bool)
                n608 = local read "单选_第13路"() -> (w102:bool)
                n609 = local read "单选_第14路"() -> (w103:bool)
                n610 = local read "单选_第15路"() -> (w104:bool)
                n611 = local read "单选_第16路"() -> (w105:bool)
                n612 = local read "输入值_1"() -> (w74:enum16{"0", "1"})
                n613 = local read "输入值_2"() -> (w75:enum16{"0", "1"})
                n614 = local read "输入值_3"() -> (w76:enum16{"0", "1"})
                n615 = local read "输入值_4"() -> (w77:enum16{"0", "1"})
                n616 = local read "输入值_5"() -> (w78:enum16{"0", "1"})
                n617 = local read "输入值_6"() -> (w79:enum16{"0", "1"})
                n618 = local read "输入值_7"() -> (w80:enum16{"0", "1"})
                n619 = local read "输入值_8"() -> (w81:enum16{"0", "1"})
                n620 = local read "输入值_9"() -> (w82:enum16{"0", "1"})
                n621 = local read "输入值_10"() -> (w83:enum16{"0", "1"})
                n622 = local read "输入值_11"() -> (w84:enum16{"0", "1"})
                n623 = local read "输入值_12"() -> (w85:enum16{"0", "1"})
                n624 = local read "输入值_13"() -> (w86:enum16{"0", "1"})
                n625 = local read "输入值_14"() -> (w87:enum16{"0", "1"})
                n626 = local read "输入值_15"() -> (w88:enum16{"0", "1"})
                n627 = local read "输入值_16"() -> (w89:enum16{"0", "1"})
                n628 = Build Array(w90, w91, w92, w93, w94, w95, w96, w97, w98, w99, w100, w101, w102, w103, w104, w105) -> (w73:bool[])
                n629 = Build Array(w74, w75, w76, w77, w78, w79, w80, w81, w82, w83, w84, w85, w86, w87, w88, w89) -> (w72:enum16{"0", "1"}[])
              }
              frame #1 {
                n630 = local read "单选_第17路"() -> (w124:bool)
                n631 = local read "单选_第18路"() -> (w125:bool)
                n632 = local read "单选_第19路"() -> (w126:bool)
                n633 = local read "单选_第20路"() -> (w127:bool)
                n634 = local read "单选_第21路"() -> (w128:bool)
                n635 = local read "单选_第22路"() -> (w129:bool)
                n636 = local read "单选_第23路"() -> (w130:bool)
                n637 = local read "单选_第24路"() -> (w131:bool)
                n638 = local read "单选_第25路"() -> (w132:bool)
                n639 = local read "单选_第26路"() -> (w133:bool)
                n640 = local read "单选_第27路"() -> (w134:bool)
                n641 = local read "单选_第28路"() -> (w135:bool)
                n642 = local read "单选_第29路"() -> (w136:bool)
                n643 = local read "单选_第30路"() -> (w137:bool)
                n644 = local read "单选_第31路"() -> (w138:bool)
                n645 = local read "单选_第32路"() -> (w139:bool)
                n646 = local read "输入值_17"() -> (w108:enum16{"0", "1"})
                n647 = local read "输入值_18"() -> (w109:enum16{"0", "1"})
                n648 = local read "输入值_19"() -> (w110:enum16{"0", "1"})
                n649 = local read "输入值_20"() -> (w111:enum16{"0", "1"})
                n650 = local read "输入值_21"() -> (w112:enum16{"0", "1"})
                n651 = local read "输入值_22"() -> (w113:enum16{"0", "1"})
                n652 = local read "输入值_23"() -> (w114:enum16{"0", "1"})
                n653 = local read "输入值_24"() -> (w115:enum16{"0", "1"})
                n654 = local read "输入值_25"() -> (w116:enum16{"0", "1"})
                n655 = local read "输入值_26"() -> (w117:enum16{"0", "1"})
                n656 = local read "输入值_27"() -> (w118:enum16{"0", "1"})
                n657 = local read "输入值_28"() -> (w119:enum16{"0", "1"})
                n658 = local read "输入值_29"() -> (w120:enum16{"0", "1"})
                n659 = local read "输入值_30"() -> (w121:enum16{"0", "1"})
                n660 = local read "输入值_31"() -> (w122:enum16{"0", "1"})
                n661 = local read "输入值_32"() -> (w123:enum16{"0", "1"})
                n662 = Build Array(w124, w125, w126, w127, w128, w129, w130, w131, w132, w133, w134, w135, w136, w137, w138, w139) -> (w107:bool[])
                n663 = Build Array(w108, w109, w110, w111, w112, w113, w114, w115, w116, w117, w118, w119, w120, w121, w122, w123) -> (w106:enum16{"0", "1"}[])
              }
              frame #2 {
                n664 = local read "单选_第33路"() -> (w158:bool)
                n665 = local read "单选_第34路"() -> (w159:bool)
                n666 = local read "单选_第35路"() -> (w160:bool)
                n667 = local read "单选_第36路"() -> (w161:bool)
                n668 = local read "单选_第37路"() -> (w162:bool)
                n669 = local read "单选_第38路"() -> (w163:bool)
                n670 = local read "单选_第39路"() -> (w164:bool)
                n671 = local read "单选_第40路"() -> (w165:bool)
                n672 = local read "单选_第41路"() -> (w166:bool)
                n673 = local read "单选_第42路"() -> (w167:bool)
                n674 = local read "单选_第43路"() -> (w168:bool)
                n675 = local read "单选_第44路"() -> (w169:bool)
                n676 = local read "单选_第45路"() -> (w170:bool)
                n677 = local read "单选_第46路"() -> (w171:bool)
                n678 = local read "单选_第47路"() -> (w172:bool)
                n679 = local read "单选_第48路"() -> (w173:bool)
                n680 = local read "输入值_33"() -> (w142:enum16{"0", "1"})
                n681 = local read "输入值_34"() -> (w143:enum16{"0", "1"})
                n682 = local read "输入值_35"() -> (w144:enum16{"0", "1"})
                n683 = local read "输入值_36"() -> (w145:enum16{"0", "1"})
                n684 = local read "输入值_37"() -> (w146:enum16{"0", "1"})
                n685 = local read "输入值_38"() -> (w147:enum16{"0", "1"})
                n686 = local read "输入值_39"() -> (w148:enum16{"0", "1"})
                n687 = local read "输入值_40"() -> (w149:enum16{"0", "1"})
                n688 = local read "输入值_41"() -> (w150:enum16{"0", "1"})
                n689 = local read "输入值_42"() -> (w151:enum16{"0", "1"})
                n690 = local read "输入值_43"() -> (w152:enum16{"0", "1"})
                n691 = local read "输入值_44"() -> (w153:enum16{"0", "1"})
                n692 = local read "输入值_45"() -> (w154:enum16{"0", "1"})
                n693 = local read "输入值_46"() -> (w155:enum16{"0", "1"})
                n694 = local read "输入值_47"() -> (w156:enum16{"0", "1"})
                n695 = local read "输入值_48"() -> (w157:enum16{"0", "1"})
                n696 = Build Array(w142, w143, w144, w145, w146, w147, w148, w149, w150, w151, w152, w153, w154, w155, w156, w157) -> (w140:enum16{"0", "1"}[])
                n697 = Build Array(w158, w159, w160, w161, w162, w163, w164, w165, w166, w167, w168, w169, w170, w171, w172, w173) -> (w141:bool[])
              }
              frame #3 {
                n698 = local read "单选_第49路"() -> (w192:bool)
                n699 = local read "单选_第50路"() -> (w193:bool)
                n700 = local read "单选_第51路"() -> (w194:bool)
                n701 = local read "单选_第52路"() -> (w195:bool)
                n702 = local read "单选_第53路"() -> (w196:bool)
                n703 = local read "单选_第54路"() -> (w197:bool)
                n704 = local read "单选_第55路"() -> (w198:bool)
                n705 = local read "单选_第56路"() -> (w199:bool)
                n706 = local read "单选_第57路"() -> (w200:bool)
                n707 = local read "单选_第58路"() -> (w201:bool)
                n708 = local read "单选_第59路"() -> (w202:bool)
                n709 = local read "单选_第60路"() -> (w203:bool)
                n710 = local read "单选_第61路"() -> (w204:bool)
                n711 = local read "单选_第62路"() -> (w205:bool)
                n712 = local read "单选_第63路"() -> (w206:bool)
                n713 = local read "单选_第64路"() -> (w207:bool)
                n714 = local read "输入值_49"() -> (w176:enum16{"0", "1"})
                n715 = local read "输入值_50"() -> (w177:enum16{"0", "1"})
                n716 = local read "输入值_51"() -> (w178:enum16{"0", "1"})
                n717 = local read "输入值_52"() -> (w179:enum16{"0", "1"})
                n718 = local read "输入值_53"() -> (w180:enum16{"0", "1"})
                n719 = local read "输入值_54"() -> (w181:enum16{"0", "1"})
                n720 = local read "输入值_55"() -> (w182:enum16{"0", "1"})
                n721 = local read "输入值_56"() -> (w183:enum16{"0", "1"})
                n722 = local read "输入值_57"() -> (w184:enum16{"0", "1"})
                n723 = local read "输入值_58"() -> (w185:enum16{"0", "1"})
                n724 = local read "输入值_59"() -> (w186:enum16{"0", "1"})
                n725 = local read "输入值_60"() -> (w187:enum16{"0", "1"})
                n726 = local read "输入值_61"() -> (w188:enum16{"0", "1"})
                n727 = local read "输入值_62"() -> (w189:enum16{"0", "1"})
                n728 = local read "输入值_63"() -> (w190:enum16{"0", "1"})
                n729 = local read "输入值_64"() -> (w191:enum16{"0", "1"})
                n730 = Build Array(w192, w193, w194, w195, w196, w197, w198, w199, w200, w201, w202, w203, w204, w205, w206, w207) -> (w175:bool[])
                n731 = Build Array(w176, w177, w178, w179, w180, w181, w182, w183, w184, w185, w186, w187, w188, w189, w190, w191) -> (w174:enum16{"0", "1"}[])
              }
              frame #4 {
                n732 = local read "单选_第71路"() -> (w232:bool)
                n733 = local read "单选_第79路"() -> (w240:bool)
                n734 = local read "单选_第65路"() -> (w226:bool)
                n735 = local read "单选_第66路"() -> (w227:bool)
                n736 = local read "单选_第67路"() -> (w228:bool)
                n737 = local read "单选_第68路"() -> (w229:bool)
                n738 = local read "单选_第69路"() -> (w230:bool)
                n739 = local read "单选_第70路"() -> (w231:bool)
                n740 = local read "单选_第72路"() -> (w233:bool)
                n741 = local read "单选_第73路"() -> (w234:bool)
                n742 = local read "单选_第74路"() -> (w235:bool)
                n743 = local read "单选_第75路"() -> (w236:bool)
                n744 = local read "单选_第76路"() -> (w237:bool)
                n745 = local read "单选_第77路"() -> (w238:bool)
                n746 = local read "单选_第78路"() -> (w239:bool)
                n747 = local read "单选_第80路"() -> (w241:bool)
                n748 = local read "输入值_65"() -> (w210:enum16{"0", "1"})
                n749 = local read "输入值_66"() -> (w211:enum16{"0", "1"})
                n750 = local read "输入值_67"() -> (w212:enum16{"0", "1"})
                n751 = local read "输入值_68"() -> (w213:enum16{"0", "1"})
                n752 = local read "输入值_69"() -> (w214:enum16{"0", "1"})
                n753 = local read "输入值_70"() -> (w215:enum16{"0", "1"})
                n754 = local read "输入值_71"() -> (w216:enum16{"0", "1"})
                n755 = local read "输入值_72"() -> (w217:enum16{"0", "1"})
                n756 = local read "输入值_73"() -> (w218:enum16{"0", "1"})
                n757 = local read "输入值_74"() -> (w219:enum16{"0", "1"})
                n758 = local read "输入值_75"() -> (w220:enum16{"0", "1"})
                n759 = local read "输入值_76"() -> (w221:enum16{"0", "1"})
                n760 = local read "输入值_77"() -> (w222:enum16{"0", "1"})
                n761 = local read "输入值_78"() -> (w223:enum16{"0", "1"})
                n762 = local read "输入值_79"() -> (w224:enum16{"0", "1"})
                n763 = local read "输入值_80"() -> (w225:enum16{"0", "1"})
                n764 = Build Array(w210, w211, w212, w213, w214, w215, w216, w217, w218, w219, w220, w221, w222, w223, w224, w225) -> (w208:enum16{"0", "1"}[])
                n765 = Build Array(w226, w227, w228, w229, w230, w231, w232, w233, w234, w235, w236, w237, w238, w239, w240, w241) -> (w209:bool[])
              }
            }
            n766 = local read "数组_输入值"() -> (w70:enum16{"0", "1"}[])
            n767 = local read "数组_选择?"() -> (w71:bool[])
            n768 = local write "测试结论"("") -> ()
            n769 = local write "同步_A1"(w68) -> ()
            n770 = local write "同步_A2"(w68) -> ()
            n771 = Insert Into Array(array=w70, index=0 ("索引 (行)"), new element #1=w59, new element #2=w58, new element #3=w57, new element #4=w56, new element #5=w55) -> (w69:enum16{"0", "1"}[])
            n772 = Insert Into Array(array=w71, index=0 ("索引 (行)"), new element #1=w65, new element #2=w64, new element #3=w63, new element #4=w62, new element #5=w61) -> (w54:bool[])
            n773 = local write "数组_输入值"(w69) -> ()
            n774 = local write "数组_选择?"(w54) -> ()
            n775 = Or Array Elements(Boolean array=w54) -> ()  [unwired: 1 out]
          }
          frame #1 {
            w243 = cluster{u32, u32}[] [{9868950, 9868950}]
            n776 = property on="light_1" class="Bool (严格)"("Colors [4]"=w243) -> ()  [unwired: 2 in, 2 out]
            n777 = property on="light_2" class="Bool (严格)"("Colors [4]"=w243) -> ()  [unwired: 2 in, 2 out]
            n778 = property on="light_3" class="Bool (严格)"("Colors [4]"=w243) -> ()  [unwired: 2 in, 2 out]
            n779 = property on="light_4" class="Bool (严格)"("Colors [4]"=w243) -> ()  [unwired: 2 in, 2 out]
            n780 = property on="light_5" class="Bool (严格)"("Colors [4]"=w243) -> ()  [unwired: 2 in, 2 out]
            n781 = property on="light_6" class="Bool (严格)"("Colors [4]"=w243) -> ()  [unwired: 2 in, 2 out]
            n782 = property on="light_7" class="Bool (严格)"("Colors [4]"=w243) -> ()  [unwired: 2 in, 2 out]
            n783 = property on="light_8" class="Bool (严格)"("Colors [4]"=w243) -> ()  [unwired: 2 in, 2 out]
            n784 = property on="light_9" class="Bool (严格)"("Colors [4]"=w243) -> ()  [unwired: 2 in, 2 out]
            n785 = property on="light_10" class="Bool (严格)"("Colors [4]"=w243) -> ()  [unwired: 2 in, 2 out]
            n786 = property on="light_11" class="Bool (严格)"("Colors [4]"=w243) -> ()  [unwired: 2 in, 2 out]
            n787 = property on="light_12" class="Bool (严格)"("Colors [4]"=w243) -> ()  [unwired: 2 in, 2 out]
            n788 = property on="light_13" class="Bool (严格)"("Colors [4]"=w243) -> ()  [unwired: 2 in, 2 out]
            n789 = property on="light_14" class="Bool (严格)"("Colors [4]"=w243) -> ()  [unwired: 2 in, 2 out]
            n790 = property on="light_15" class="Bool (严格)"("Colors [4]"=w243) -> ()  [unwired: 2 in, 2 out]
            n791 = property on="light_16" class="Bool (严格)"("Colors [4]"=w243) -> ()  [unwired: 2 in, 2 out]
            n792 = property on="light_17" class="Bool (严格)"("Colors [4]"=w243) -> ()  [unwired: 2 in, 2 out]
            n793 = property on="light_18" class="Bool (严格)"("Colors [4]"=w243) -> ()  [unwired: 2 in, 2 out]
            n794 = property on="light_19" class="Bool (严格)"("Colors [4]"=w243) -> ()  [unwired: 2 in, 2 out]
            n795 = property on="light_20" class="Bool (严格)"("Colors [4]"=w243) -> ()  [unwired: 2 in, 2 out]
            n796 = property on="light_21" class="Bool (严格)"("Colors [4]"=w243) -> ()  [unwired: 2 in, 2 out]
            n797 = property on="light_22" class="Bool (严格)"("Colors [4]"=w243) -> ()  [unwired: 2 in, 2 out]
            n798 = property on="light_23" class="Bool (严格)"("Colors [4]"=w243) -> ()  [unwired: 2 in, 2 out]
            n799 = property on="light_24" class="Bool (严格)"("Colors [4]"=w243) -> ()  [unwired: 2 in, 2 out]
            n800 = property on="light_25" class="Bool (严格)"("Colors [4]"=w243) -> ()  [unwired: 2 in, 2 out]
            n801 = property on="light_26" class="Bool (严格)"("Colors [4]"=w243) -> ()  [unwired: 2 in, 2 out]
            n802 = property on="light_27" class="Bool (严格)"("Colors [4]"=w243) -> ()  [unwired: 2 in, 2 out]
            n803 = property on="light_28" class="Bool (严格)"("Colors [4]"=w243) -> ()  [unwired: 2 in, 2 out]
            n804 = property on="light_29" class="Bool (严格)"("Colors [4]"=w243) -> ()  [unwired: 2 in, 2 out]
            n805 = property on="light_30" class="Bool (严格)"("Colors [4]"=w243) -> ()  [unwired: 2 in, 2 out]
            n806 = property on="light_31" class="Bool (严格)"("Colors [4]"=w243) -> ()  [unwired: 2 in, 2 out]
            n807 = property on="light_32" class="Bool (严格)"("Colors [4]"=w243) -> ()  [unwired: 2 in, 2 out]
            n808 = property on="light_33" class="Bool (严格)"("Colors [4]"=w243) -> ()  [unwired: 2 in, 2 out]
            n809 = property on="light_34" class="Bool (严格)"("Colors [4]"=w243) -> ()  [unwired: 2 in, 2 out]
            n810 = property on="light_35" class="Bool (严格)"("Colors [4]"=w243) -> ()  [unwired: 2 in, 2 out]
            n811 = property on="light_36" class="Bool (严格)"("Colors [4]"=w243) -> ()  [unwired: 2 in, 2 out]
            n812 = property on="light_37" class="Bool (严格)"("Colors [4]"=w243) -> ()  [unwired: 2 in, 2 out]
            n813 = property on="light_38" class="Bool (严格)"("Colors [4]"=w243) -> ()  [unwired: 2 in, 2 out]
            n814 = property on="light_39" class="Bool (严格)"("Colors [4]"=w243) -> ()  [unwired: 2 in, 2 out]
            n815 = property on="light_40" class="Bool (严格)"("Colors [4]"=w243) -> ()  [unwired: 2 in, 2 out]
            n816 = property on="light_41" class="Bool (严格)"("Colors [4]"=w243) -> ()  [unwired: 2 in, 2 out]
            n817 = property on="light_42" class="Bool (严格)"("Colors [4]"=w243) -> ()  [unwired: 2 in, 2 out]
            n818 = property on="light_43" class="Bool (严格)"("Colors [4]"=w243) -> ()  [unwired: 2 in, 2 out]
            n819 = property on="light_44" class="Bool (严格)"("Colors [4]"=w243) -> ()  [unwired: 2 in, 2 out]
            n820 = property on="light_45" class="Bool (严格)"("Colors [4]"=w243) -> ()  [unwired: 2 in, 2 out]
            n821 = property on="light_46" class="Bool (严格)"("Colors [4]"=w243) -> ()  [unwired: 2 in, 2 out]
            n822 = property on="light_47" class="Bool (严格)"("Colors [4]"=w243) -> ()  [unwired: 2 in, 2 out]
            n823 = property on="light_48" class="Bool (严格)"("Colors [4]"=w243) -> ()  [unwired: 2 in, 2 out]
            n824 = property on="light_49" class="Bool (严格)"("Colors [4]"=w243) -> ()  [unwired: 2 in, 2 out]
            n825 = property on="light_50" class="Bool (严格)"("Colors [4]"=w243) -> ()  [unwired: 2 in, 2 out]
            n826 = property on="light_51" class="Bool (严格)"("Colors [4]"=w243) -> ()  [unwired: 2 in, 2 out]
            n827 = property on="light_52" class="Bool (严格)"("Colors [4]"=w243) -> ()  [unwired: 2 in, 2 out]
            n828 = property on="light_53" class="Bool (严格)"("Colors [4]"=w243) -> ()  [unwired: 2 in, 2 out]
            n829 = property on="light_54" class="Bool (严格)"("Colors [4]"=w243) -> ()  [unwired: 2 in, 2 out]
            n830 = property on="light_55" class="Bool (严格)"("Colors [4]"=w243) -> ()  [unwired: 2 in, 2 out]
            n831 = property on="light_56" class="Bool (严格)"("Colors [4]"=w243) -> ()  [unwired: 2 in, 2 out]
            n832 = property on="light_57" class="Bool (严格)"("Colors [4]"=w243) -> ()  [unwired: 2 in, 2 out]
            n833 = property on="light_58" class="Bool (严格)"("Colors [4]"=w243) -> ()  [unwired: 2 in, 2 out]
            n834 = property on="light_59" class="Bool (严格)"("Colors [4]"=w243) -> ()  [unwired: 2 in, 2 out]
            n835 = property on="light_60" class="Bool (严格)"("Colors [4]"=w243) -> ()  [unwired: 2 in, 2 out]
            n836 = property on="light_61" class="Bool (严格)"("Colors [4]"=w243) -> ()  [unwired: 2 in, 2 out]
            n837 = property on="light_62" class="Bool (严格)"("Colors [4]"=w243) -> ()  [unwired: 2 in, 2 out]
            n838 = property on="light_63" class="Bool (严格)"("Colors [4]"=w243) -> ()  [unwired: 2 in, 2 out]
            n839 = property on="light_64" class="Bool (严格)"("Colors [4]"=w243) -> ()  [unwired: 2 in, 2 out]
            n840 = property on="light_65" class="Bool (严格)"("Colors [4]"=w243) -> ()  [unwired: 2 in, 2 out]
            n841 = property on="light_66" class="Bool (严格)"("Colors [4]"=w243) -> ()  [unwired: 2 in, 2 out]
            n842 = property on="light_67" class="Bool (严格)"("Colors [4]"=w243) -> ()  [unwired: 2 in, 2 out]
            n843 = property on="light_68" class="Bool (严格)"("Colors [4]"=w243) -> ()  [unwired: 2 in, 2 out]
            n844 = property on="light_69" class="Bool (严格)"("Colors [4]"=w243) -> ()  [unwired: 2 in, 2 out]
            n845 = property on="light_70" class="Bool (严格)"("Colors [4]"=w243) -> ()  [unwired: 2 in, 2 out]
            n846 = property on="light_71" class="Bool (严格)"("Colors [4]"=w243) -> ()  [unwired: 2 in, 2 out]
            n847 = property on="light_72" class="Bool (严格)"("Colors [4]"=w243) -> ()  [unwired: 2 in, 2 out]
            n848 = property on="light_73" class="Bool (严格)"("Colors [4]"=w243) -> ()  [unwired: 2 in, 2 out]
            n849 = property on="light_74" class="Bool (严格)"("Colors [4]"=w243) -> ()  [unwired: 2 in, 2 out]
            n850 = property on="light_75" class="Bool (严格)"("Colors [4]"=w243) -> ()  [unwired: 2 in, 2 out]
            n851 = property on="light_76" class="Bool (严格)"("Colors [4]"=w243) -> ()  [unwired: 2 in, 2 out]
            n852 = property on="light_77" class="Bool (严格)"("Colors [4]"=w243) -> ()  [unwired: 2 in, 2 out]
            n853 = property on="light_78" class="Bool (严格)"("Colors [4]"=w243) -> ()  [unwired: 2 in, 2 out]
            n854 = property on="light_79" class="Bool (严格)"("Colors [4]"=w243) -> ()  [unwired: 2 in, 2 out]
            n855 = property on="light_80" class="Bool (严格)"("Colors [4]"=w243) -> ()  [unwired: 2 in, 2 out]
            n856 = disable-structure shown="禁用" {
              frame Disabled {
                n857 = Initialize Array("", 16 ("维数大小"), 4 ("维数大小")) -> (w247:string[][])
                n858 = local write "D_IN_1"(w247) -> ()
                n859 = local write "D_IN_2"(w247) -> ()
                n860 = local write "D_IN_3"(w247) -> ()
                n861 = local write "D_IN_4"(w247) -> ()
                n862 = local write "D_IN_5"(w247) -> ()
              }
              frame Enabled {
              }
            }
            n863 = property on="btn_关闭" class="Bool"("DisabledEnum"=T1."Disabled and Grayed Out" ("禁用")) -> ()  [unwired: 2 in, 2 out]
          }
          frame #2 {
            w248 = 0 ("同步_A1")
            n864 = local read "数组_选择?"() -> (w254:bool[])
            n865 = Or Array Elements(Boolean array=w254) -> (logical OR=w253:bool)
            n866 = case shown="真" w253 {
              frame False {
                n867 = call "显示对话框信息"("Message"="请选择数字量输入路数") -> ()  [unwired: 9 in, 2 out]
              }
              frame True {
                w257 = "DIStart" ("名称（未命名）")
                n868 = Obtain Notifier(name (unnamed)=w257, notification data type=w257) -> (notifier out=w256:refnum<notifier>)  [unwired: 2 in, 2 out]
                n869 = Send Notification(notification="DInput" ("通知"), notifier=w256) -> ()  [unwired: 1 in, 2 out]
              }
            }
            n870 = local write "第几组数据"(0 ("第几组数据")) -> ()
            n871 = local write "同步_A1"(w248) -> ()
            n872 = local write "同步_A2"(w248) -> ()
            n873 = Initialize Array(FALSE, 80 ("维数大小")) -> (w250:bool[])
            n874 = local write "合格？"(w250) -> ()
          }
        }
      }
      event "btn_全选": Value Change {
        w259 = TRUE ("单选_第41路")
        n875 = event-data() -> ()  [unwired: 1 in, 5 out]
        n876 = local write "单选_第1路"(w259) -> ()
        n877 = local write "单选_第2路"(w259) -> ()
        n878 = local write "单选_第3路"(w259) -> ()
        n879 = local write "单选_第4路"(w259) -> ()
        n880 = local write "单选_第5路"(w259) -> ()
        n881 = local write "单选_第6路"(w259) -> ()
        n882 = local write "单选_第7路"(w259) -> ()
        n883 = local write "单选_第8路"(w259) -> ()
        n884 = local write "单选_第9路"(w259) -> ()
        n885 = local write "单选_第10路"(w259) -> ()
        n886 = local write "单选_第11路"(w259) -> ()
        n887 = local write "单选_第12路"(w259) -> ()
        n888 = local write "单选_第13路"(w259) -> ()
        n889 = local write "单选_第14路"(w259) -> ()
        n890 = local write "单选_第15路"(w259) -> ()
        n891 = local write "单选_第16路"(w259) -> ()
        n892 = local write "单选_第17路"(w259) -> ()
        n893 = local write "单选_第18路"(w259) -> ()
        n894 = local write "单选_第19路"(w259) -> ()
        n895 = local write "单选_第20路"(w259) -> ()
        n896 = local write "单选_第21路"(w259) -> ()
        n897 = local write "单选_第22路"(w259) -> ()
        n898 = local write "单选_第23路"(w259) -> ()
        n899 = local write "单选_第24路"(w259) -> ()
        n900 = local write "单选_第25路"(w259) -> ()
        n901 = local write "单选_第26路"(w259) -> ()
        n902 = local write "单选_第27路"(w259) -> ()
        n903 = local write "单选_第28路"(w259) -> ()
        n904 = local write "单选_第29路"(w259) -> ()
        n905 = local write "单选_第30路"(w259) -> ()
        n906 = local write "单选_第31路"(w259) -> ()
        n907 = local write "单选_第32路"(w259) -> ()
        n908 = local write "单选_第33路"(w259) -> ()
        n909 = local write "单选_第34路"(w259) -> ()
        n910 = local write "单选_第35路"(w259) -> ()
        n911 = local write "单选_第36路"(w259) -> ()
        n912 = local write "单选_第37路"(w259) -> ()
        n913 = local write "单选_第38路"(w259) -> ()
        n914 = local write "单选_第39路"(w259) -> ()
        n915 = local write "单选_第40路"(w259) -> ()
        n916 = local write "单选_第41路"(w259) -> ()
        n917 = local write "单选_第42路"(w259) -> ()
        n918 = local write "单选_第43路"(w259) -> ()
        n919 = local write "单选_第44路"(w259) -> ()
        n920 = local write "单选_第45路"(w259) -> ()
        n921 = local write "单选_第46路"(w259) -> ()
        n922 = local write "单选_第47路"(w259) -> ()
        n923 = local write "单选_第48路"(w259) -> ()
        n924 = local write "单选_第49路"(w259) -> ()
        n925 = local write "单选_第50路"(w259) -> ()
        n926 = local write "单选_第51路"(w259) -> ()
        n927 = local write "单选_第52路"(w259) -> ()
        n928 = local write "单选_第53路"(w259) -> ()
        n929 = local write "单选_第54路"(w259) -> ()
        n930 = local write "单选_第55路"(w259) -> ()
        n931 = local write "单选_第56路"(w259) -> ()
        n932 = local write "单选_第57路"(w259) -> ()
        n933 = local write "单选_第58路"(w259) -> ()
        n934 = local write "单选_第59路"(w259) -> ()
        n935 = local write "单选_第60路"(w259) -> ()
        n936 = local write "单选_第61路"(w259) -> ()
        n937 = local write "单选_第62路"(w259) -> ()
        n938 = local write "单选_第63路"(w259) -> ()
        n939 = local write "单选_第64路"(w259) -> ()
        n940 = local write "单选_第71路"(w259) -> ()
        n941 = local write "单选_第79路"(w259) -> ()
        n942 = local write "单选_第65路"(w259) -> ()
        n943 = local write "单选_第66路"(w259) -> ()
        n944 = local write "单选_第67路"(w259) -> ()
        n945 = local write "单选_第68路"(w259) -> ()
        n946 = local write "单选_第69路"(w259) -> ()
        n947 = local write "单选_第70路"(w259) -> ()
        n948 = local write "单选_第72路"(w259) -> ()
        n949 = local write "单选_第73路"(w259) -> ()
        n950 = local write "单选_第74路"(w259) -> ()
        n951 = local write "单选_第75路"(w259) -> ()
        n952 = local write "单选_第76路"(w259) -> ()
        n953 = local write "单选_第77路"(w259) -> ()
        n954 = local write "单选_第78路"(w259) -> ()
        n955 = local write "单选_第80路"(w259) -> ()
      }
      event "btn_反选": Value Change {
        n956 = event-data() -> ()  [unwired: 1 in, 5 out]
        n957 = local read "单选_第1路"() -> (w419:bool)
        n958 = local read "单选_第2路"() -> (w417:bool)
        n959 = local read "单选_第3路"() -> (w415:bool)
        n960 = local read "单选_第4路"() -> (w413:bool)
        n961 = local read "单选_第5路"() -> (w411:bool)
        n962 = local read "单选_第6路"() -> (w409:bool)
        n963 = local read "单选_第7路"() -> (w408:bool)
        n964 = local read "单选_第8路"() -> (w407:bool)
        n965 = local read "单选_第9路"() -> (w406:bool)
        n966 = local read "单选_第10路"() -> (w405:bool)
        n967 = local read "单选_第11路"() -> (w404:bool)
        n968 = local read "单选_第12路"() -> (w403:bool)
        n969 = local read "单选_第13路"() -> (w402:bool)
        n970 = local read "单选_第14路"() -> (w401:bool)
        n971 = local read "单选_第15路"() -> (w400:bool)
        n972 = local read "单选_第16路"() -> (w399:bool)
        n973 = local read "单选_第17路"() -> (w398:bool)
        n974 = local read "单选_第18路"() -> (w397:bool)
        n975 = local read "单选_第19路"() -> (w396:bool)
        n976 = local read "单选_第20路"() -> (w395:bool)
        n977 = local read "单选_第21路"() -> (w394:bool)
        n978 = local read "单选_第22路"() -> (w393:bool)
        n979 = local read "单选_第23路"() -> (w392:bool)
        n980 = local read "单选_第24路"() -> (w391:bool)
        n981 = local read "单选_第25路"() -> (w390:bool)
        n982 = local read "单选_第26路"() -> (w389:bool)
        n983 = local read "单选_第27路"() -> (w388:bool)
        n984 = local read "单选_第28路"() -> (w387:bool)
        n985 = local read "单选_第29路"() -> (w386:bool)
        n986 = local read "单选_第30路"() -> (w385:bool)
        n987 = local read "单选_第31路"() -> (w384:bool)
        n988 = local read "单选_第32路"() -> (w383:bool)
        n989 = local read "单选_第33路"() -> (w382:bool)
        n990 = local read "单选_第34路"() -> (w381:bool)
        n991 = local read "单选_第35路"() -> (w380:bool)
        n992 = local read "单选_第36路"() -> (w379:bool)
        n993 = local read "单选_第37路"() -> (w378:bool)
        n994 = local read "单选_第38路"() -> (w377:bool)
        n995 = local read "单选_第39路"() -> (w376:bool)
        n996 = local read "单选_第40路"() -> (w375:bool)
        n997 = Not(x=w419) -> (.not. x?=w418:bool)
        n998 = Not(x=w417) -> (.not. x?=w416:bool)
        n999 = Not(x=w415) -> (.not. x?=w414:bool)
        n1000 = Not(x=w413) -> (.not. x?=w412:bool)
        n1001 = Not(x=w411) -> (.not. x?=w410:bool)
        n1002 = Not(x=w409) -> (.not. x?=w374:bool)
        n1003 = Not(x=w408) -> (.not. x?=w373:bool)
        n1004 = Not(x=w407) -> (.not. x?=w372:bool)
        n1005 = Not(x=w406) -> (.not. x?=w371:bool)
        n1006 = Not(x=w405) -> (.not. x?=w370:bool)
        n1007 = Not(x=w404) -> (.not. x?=w369:bool)
        n1008 = Not(x=w403) -> (.not. x?=w368:bool)
        n1009 = Not(x=w402) -> (.not. x?=w367:bool)
        n1010 = Not(x=w401) -> (.not. x?=w366:bool)
        n1011 = Not(x=w400) -> (.not. x?=w365:bool)
        n1012 = Not(x=w399) -> (.not. x?=w364:bool)
        n1013 = Not(x=w398) -> (.not. x?=w363:bool)
        n1014 = Not(x=w397) -> (.not. x?=w362:bool)
        n1015 = Not(x=w396) -> (.not. x?=w361:bool)
        n1016 = Not(x=w395) -> (.not. x?=w360:bool)
        n1017 = Not(x=w394) -> (.not. x?=w359:bool)
        n1018 = Not(x=w393) -> (.not. x?=w358:bool)
        n1019 = Not(x=w392) -> (.not. x?=w357:bool)
        n1020 = Not(x=w391) -> (.not. x?=w356:bool)
        n1021 = Not(x=w390) -> (.not. x?=w355:bool)
        n1022 = Not(x=w389) -> (.not. x?=w354:bool)
        n1023 = Not(x=w388) -> (.not. x?=w353:bool)
        n1024 = Not(x=w387) -> (.not. x?=w352:bool)
        n1025 = Not(x=w386) -> (.not. x?=w351:bool)
        n1026 = Not(x=w385) -> (.not. x?=w350:bool)
        n1027 = Not(x=w384) -> (.not. x?=w349:bool)
        n1028 = Not(x=w383) -> (.not. x?=w348:bool)
        n1029 = Not(x=w382) -> (.not. x?=w347:bool)
        n1030 = Not(x=w381) -> (.not. x?=w346:bool)
        n1031 = Not(x=w380) -> (.not. x?=w345:bool)
        n1032 = Not(x=w379) -> (.not. x?=w344:bool)
        n1033 = Not(x=w378) -> (.not. x?=w343:bool)
        n1034 = Not(x=w377) -> (.not. x?=w342:bool)
        n1035 = Not(x=w376) -> (.not. x?=w341:bool)
        n1036 = Not(x=w375) -> (.not. x?=w340:bool)
        n1037 = local write "单选_第1路"(w418) -> ()
        n1038 = local write "单选_第2路"(w416) -> ()
        n1039 = local write "单选_第3路"(w414) -> ()
        n1040 = local write "单选_第4路"(w412) -> ()
        n1041 = local write "单选_第5路"(w410) -> ()
        n1042 = local write "单选_第6路"(w374) -> ()
        n1043 = local write "单选_第7路"(w373) -> ()
        n1044 = local write "单选_第8路"(w372) -> ()
        n1045 = local write "单选_第9路"(w371) -> ()
        n1046 = local write "单选_第10路"(w370) -> ()
        n1047 = local write "单选_第11路"(w369) -> ()
        n1048 = local write "单选_第12路"(w368) -> ()
        n1049 = local write "单选_第13路"(w367) -> ()
        n1050 = local write "单选_第14路"(w366) -> ()
        n1051 = local write "单选_第15路"(w365) -> ()
        n1052 = local write "单选_第16路"(w364) -> ()
        n1053 = local write "单选_第17路"(w363) -> ()
        n1054 = local write "单选_第18路"(w362) -> ()
        n1055 = local write "单选_第19路"(w361) -> ()
        n1056 = local write "单选_第20路"(w360) -> ()
        n1057 = local write "单选_第21路"(w359) -> ()
        n1058 = local write "单选_第22路"(w358) -> ()
        n1059 = local write "单选_第23路"(w357) -> ()
        n1060 = local write "单选_第24路"(w356) -> ()
        n1061 = local write "单选_第25路"(w355) -> ()
        n1062 = local write "单选_第26路"(w354) -> ()
        n1063 = local write "单选_第27路"(w353) -> ()
        n1064 = local write "单选_第28路"(w352) -> ()
        n1065 = local write "单选_第29路"(w351) -> ()
        n1066 = local write "单选_第30路"(w350) -> ()
        n1067 = local write "单选_第31路"(w349) -> ()
        n1068 = local write "单选_第32路"(w348) -> ()
        n1069 = local write "单选_第33路"(w347) -> ()
        n1070 = local write "单选_第34路"(w346) -> ()
        n1071 = local write "单选_第35路"(w345) -> ()
        n1072 = local write "单选_第36路"(w344) -> ()
        n1073 = local write "单选_第37路"(w343) -> ()
        n1074 = local write "单选_第38路"(w342) -> ()
        n1075 = local write "单选_第39路"(w341) -> ()
        n1076 = local write "单选_第40路"(w340) -> ()
        n1077 = local read "单选_第71路"() -> (w309:bool)
        n1078 = local read "单选_第79路"() -> (w301:bool)
        n1079 = local read "单选_第41路"() -> (w339:bool)
        n1080 = local read "单选_第42路"() -> (w338:bool)
        n1081 = local read "单选_第43路"() -> (w337:bool)
        n1082 = local read "单选_第44路"() -> (w336:bool)
        n1083 = local read "单选_第45路"() -> (w335:bool)
        n1084 = local read "单选_第46路"() -> (w334:bool)
        n1085 = local read "单选_第47路"() -> (w333:bool)
        n1086 = local read "单选_第48路"() -> (w332:bool)
        n1087 = local read "单选_第49路"() -> (w331:bool)
        n1088 = local read "单选_第50路"() -> (w330:bool)
        n1089 = local read "单选_第51路"() -> (w329:bool)
        n1090 = local read "单选_第52路"() -> (w328:bool)
        n1091 = local read "单选_第53路"() -> (w327:bool)
        n1092 = local read "单选_第54路"() -> (w326:bool)
        n1093 = local read "单选_第55路"() -> (w325:bool)
        n1094 = local read "单选_第56路"() -> (w324:bool)
        n1095 = local read "单选_第57路"() -> (w323:bool)
        n1096 = local read "单选_第58路"() -> (w322:bool)
        n1097 = local read "单选_第59路"() -> (w321:bool)
        n1098 = local read "单选_第60路"() -> (w320:bool)
        n1099 = local read "单选_第61路"() -> (w319:bool)
        n1100 = local read "单选_第62路"() -> (w318:bool)
        n1101 = local read "单选_第63路"() -> (w317:bool)
        n1102 = local read "单选_第64路"() -> (w316:bool)
        n1103 = local read "单选_第65路"() -> (w315:bool)
        n1104 = local read "单选_第66路"() -> (w314:bool)
        n1105 = local read "单选_第67路"() -> (w313:bool)
        n1106 = local read "单选_第68路"() -> (w312:bool)
        n1107 = local read "单选_第69路"() -> (w311:bool)
        n1108 = local read "单选_第70路"() -> (w310:bool)
        n1109 = local read "单选_第72路"() -> (w308:bool)
        n1110 = local read "单选_第73路"() -> (w307:bool)
        n1111 = local read "单选_第74路"() -> (w306:bool)
        n1112 = local read "单选_第75路"() -> (w305:bool)
        n1113 = local read "单选_第76路"() -> (w304:bool)
        n1114 = local read "单选_第77路"() -> (w303:bool)
        n1115 = local read "单选_第78路"() -> (w302:bool)
        n1116 = local read "单选_第80路"() -> (w300:bool)
        n1117 = Not(x=w339) -> (.not. x?=w299:bool)
        n1118 = Not(x=w338) -> (.not. x?=w298:bool)
        n1119 = Not(x=w337) -> (.not. x?=w297:bool)
        n1120 = Not(x=w336) -> (.not. x?=w296:bool)
        n1121 = Not(x=w335) -> (.not. x?=w295:bool)
        n1122 = Not(x=w334) -> (.not. x?=w294:bool)
        n1123 = Not(x=w333) -> (.not. x?=w293:bool)
        n1124 = Not(x=w332) -> (.not. x?=w292:bool)
        n1125 = Not(x=w331) -> (.not. x?=w291:bool)
        n1126 = Not(x=w330) -> (.not. x?=w290:bool)
        n1127 = Not(x=w329) -> (.not. x?=w289:bool)
        n1128 = Not(x=w328) -> (.not. x?=w288:bool)
        n1129 = Not(x=w327) -> (.not. x?=w287:bool)
        n1130 = Not(x=w326) -> (.not. x?=w286:bool)
        n1131 = Not(x=w325) -> (.not. x?=w285:bool)
        n1132 = Not(x=w324) -> (.not. x?=w284:bool)
        n1133 = Not(x=w323) -> (.not. x?=w283:bool)
        n1134 = Not(x=w322) -> (.not. x?=w282:bool)
        n1135 = Not(x=w321) -> (.not. x?=w281:bool)
        n1136 = Not(x=w320) -> (.not. x?=w280:bool)
        n1137 = Not(x=w319) -> (.not. x?=w279:bool)
        n1138 = Not(x=w318) -> (.not. x?=w278:bool)
        n1139 = Not(x=w317) -> (.not. x?=w277:bool)
        n1140 = Not(x=w316) -> (.not. x?=w276:bool)
        n1141 = Not(x=w315) -> (.not. x?=w275:bool)
        n1142 = Not(x=w314) -> (.not. x?=w274:bool)
        n1143 = Not(x=w313) -> (.not. x?=w273:bool)
        n1144 = Not(x=w312) -> (.not. x?=w272:bool)
        n1145 = Not(x=w311) -> (.not. x?=w271:bool)
        n1146 = Not(x=w310) -> (.not. x?=w270:bool)
        n1147 = Not(x=w309) -> (.not. x?=w269:bool)
        n1148 = Not(x=w308) -> (.not. x?=w268:bool)
        n1149 = Not(x=w307) -> (.not. x?=w267:bool)
        n1150 = Not(x=w306) -> (.not. x?=w266:bool)
        n1151 = Not(x=w305) -> (.not. x?=w265:bool)
        n1152 = Not(x=w304) -> (.not. x?=w264:bool)
        n1153 = Not(x=w303) -> (.not. x?=w263:bool)
        n1154 = Not(x=w302) -> (.not. x?=w262:bool)
        n1155 = Not(x=w301) -> (.not. x?=w261:bool)
        n1156 = Not(x=w300) -> (.not. x?=w260:bool)
        n1157 = local write "单选_第71路"(w269) -> ()
        n1158 = local write "单选_第79路"(w261) -> ()
        n1159 = local write "单选_第41路"(w299) -> ()
        n1160 = local write "单选_第42路"(w298) -> ()
        n1161 = local write "单选_第43路"(w297) -> ()
        n1162 = local write "单选_第44路"(w296) -> ()
        n1163 = local write "单选_第45路"(w295) -> ()
        n1164 = local write "单选_第46路"(w294) -> ()
        n1165 = local write "单选_第47路"(w293) -> ()
        n1166 = local write "单选_第48路"(w292) -> ()
        n1167 = local write "单选_第49路"(w291) -> ()
        n1168 = local write "单选_第50路"(w290) -> ()
        n1169 = local write "单选_第51路"(w289) -> ()
        n1170 = local write "单选_第52路"(w288) -> ()
        n1171 = local write "单选_第53路"(w287) -> ()
        n1172 = local write "单选_第54路"(w286) -> ()
        n1173 = local write "单选_第55路"(w285) -> ()
        n1174 = local write "单选_第56路"(w284) -> ()
        n1175 = local write "单选_第57路"(w283) -> ()
        n1176 = local write "单选_第58路"(w282) -> ()
        n1177 = local write "单选_第59路"(w281) -> ()
        n1178 = local write "单选_第60路"(w280) -> ()
        n1179 = local write "单选_第61路"(w279) -> ()
        n1180 = local write "单选_第62路"(w278) -> ()
        n1181 = local write "单选_第63路"(w277) -> ()
        n1182 = local write "单选_第64路"(w276) -> ()
        n1183 = local write "单选_第65路"(w275) -> ()
        n1184 = local write "单选_第66路"(w274) -> ()
        n1185 = local write "单选_第67路"(w273) -> ()
        n1186 = local write "单选_第68路"(w272) -> ()
        n1187 = local write "单选_第69路"(w271) -> ()
        n1188 = local write "单选_第70路"(w270) -> ()
        n1189 = local write "单选_第72路"(w268) -> ()
        n1190 = local write "单选_第73路"(w267) -> ()
        n1191 = local write "单选_第74路"(w266) -> ()
        n1192 = local write "单选_第75路"(w265) -> ()
        n1193 = local write "单选_第76路"(w264) -> ()
        n1194 = local write "单选_第77路"(w263) -> ()
        n1195 = local write "单选_第78路"(w262) -> ()
        n1196 = local write "单选_第80路"(w260) -> ()
      }
      event "btn_置1": Value Change {
        w420 = enum16{"0", "1"}."1" ("输入值_41")
        n1197 = event-data() -> ()  [unwired: 1 in, 5 out]
        n1198 = local write "输入值_1"(w420) -> ()
        n1199 = local write "输入值_2"(w420) -> ()
        n1200 = local write "输入值_3"(w420) -> ()
        n1201 = local write "输入值_4"(w420) -> ()
        n1202 = local write "输入值_5"(w420) -> ()
        n1203 = local write "输入值_6"(w420) -> ()
        n1204 = local write "输入值_7"(w420) -> ()
        n1205 = local write "输入值_8"(w420) -> ()
        n1206 = local write "输入值_9"(w420) -> ()
        n1207 = local write "输入值_10"(w420) -> ()
        n1208 = local write "输入值_11"(w420) -> ()
        n1209 = local write "输入值_12"(w420) -> ()
        n1210 = local write "输入值_13"(w420) -> ()
        n1211 = local write "输入值_14"(w420) -> ()
        n1212 = local write "输入值_15"(w420) -> ()
        n1213 = local write "输入值_16"(w420) -> ()
        n1214 = local write "输入值_17"(w420) -> ()
        n1215 = local write "输入值_18"(w420) -> ()
        n1216 = local write "输入值_19"(w420) -> ()
        n1217 = local write "输入值_20"(w420) -> ()
        n1218 = local write "输入值_21"(w420) -> ()
        n1219 = local write "输入值_22"(w420) -> ()
        n1220 = local write "输入值_23"(w420) -> ()
        n1221 = local write "输入值_24"(w420) -> ()
        n1222 = local write "输入值_25"(w420) -> ()
        n1223 = local write "输入值_26"(w420) -> ()
        n1224 = local write "输入值_27"(w420) -> ()
        n1225 = local write "输入值_28"(w420) -> ()
        n1226 = local write "输入值_29"(w420) -> ()
        n1227 = local write "输入值_30"(w420) -> ()
        n1228 = local write "输入值_31"(w420) -> ()
        n1229 = local write "输入值_32"(w420) -> ()
        n1230 = local write "输入值_33"(w420) -> ()
        n1231 = local write "输入值_34"(w420) -> ()
        n1232 = local write "输入值_35"(w420) -> ()
        n1233 = local write "输入值_36"(w420) -> ()
        n1234 = local write "输入值_37"(w420) -> ()
        n1235 = local write "输入值_38"(w420) -> ()
        n1236 = local write "输入值_39"(w420) -> ()
        n1237 = local write "输入值_40"(w420) -> ()
        n1238 = local write "输入值_41"(w420) -> ()
        n1239 = local write "输入值_42"(w420) -> ()
        n1240 = local write "输入值_43"(w420) -> ()
        n1241 = local write "输入值_44"(w420) -> ()
        n1242 = local write "输入值_45"(w420) -> ()
        n1243 = local write "输入值_46"(w420) -> ()
        n1244 = local write "输入值_47"(w420) -> ()
        n1245 = local write "输入值_48"(w420) -> ()
        n1246 = local write "输入值_49"(w420) -> ()
        n1247 = local write "输入值_50"(w420) -> ()
        n1248 = local write "输入值_51"(w420) -> ()
        n1249 = local write "输入值_52"(w420) -> ()
        n1250 = local write "输入值_53"(w420) -> ()
        n1251 = local write "输入值_54"(w420) -> ()
        n1252 = local write "输入值_55"(w420) -> ()
        n1253 = local write "输入值_56"(w420) -> ()
        n1254 = local write "输入值_57"(w420) -> ()
        n1255 = local write "输入值_58"(w420) -> ()
        n1256 = local write "输入值_59"(w420) -> ()
        n1257 = local write "输入值_60"(w420) -> ()
        n1258 = local write "输入值_61"(w420) -> ()
        n1259 = local write "输入值_62"(w420) -> ()
        n1260 = local write "输入值_63"(w420) -> ()
        n1261 = local write "输入值_64"(w420) -> ()
        n1262 = local write "输入值_65"(w420) -> ()
        n1263 = local write "输入值_66"(w420) -> ()
        n1264 = local write "输入值_67"(w420) -> ()
        n1265 = local write "输入值_68"(w420) -> ()
        n1266 = local write "输入值_69"(w420) -> ()
        n1267 = local write "输入值_70"(w420) -> ()
        n1268 = local write "输入值_71"(w420) -> ()
        n1269 = local write "输入值_72"(w420) -> ()
        n1270 = local write "输入值_73"(w420) -> ()
        n1271 = local write "输入值_74"(w420) -> ()
        n1272 = local write "输入值_75"(w420) -> ()
        n1273 = local write "输入值_76"(w420) -> ()
        n1274 = local write "输入值_77"(w420) -> ()
        n1275 = local write "输入值_78"(w420) -> ()
        n1276 = local write "输入值_79"(w420) -> ()
        n1277 = local write "输入值_80"(w420) -> ()
      }
      event "btn_置0": Value Change {
        w421 = enum16{"0", "1"}."0" ("输入值_41")
        n1278 = event-data() -> ()  [unwired: 1 in, 5 out]
        n1279 = local write "输入值_1"(w421) -> ()
        n1280 = local write "输入值_2"(w421) -> ()
        n1281 = local write "输入值_3"(w421) -> ()
        n1282 = local write "输入值_4"(w421) -> ()
        n1283 = local write "输入值_5"(w421) -> ()
        n1284 = local write "输入值_6"(w421) -> ()
        n1285 = local write "输入值_7"(w421) -> ()
        n1286 = local write "输入值_8"(w421) -> ()
        n1287 = local write "输入值_9"(w421) -> ()
        n1288 = local write "输入值_10"(w421) -> ()
        n1289 = local write "输入值_11"(w421) -> ()
        n1290 = local write "输入值_12"(w421) -> ()
        n1291 = local write "输入值_13"(w421) -> ()
        n1292 = local write "输入值_14"(w421) -> ()
        n1293 = local write "输入值_15"(w421) -> ()
        n1294 = local write "输入值_16"(w421) -> ()
        n1295 = local write "输入值_17"(w421) -> ()
        n1296 = local write "输入值_18"(w421) -> ()
        n1297 = local write "输入值_19"(w421) -> ()
        n1298 = local write "输入值_20"(w421) -> ()
        n1299 = local write "输入值_21"(w421) -> ()
        n1300 = local write "输入值_22"(w421) -> ()
        n1301 = local write "输入值_23"(w421) -> ()
        n1302 = local write "输入值_24"(w421) -> ()
        n1303 = local write "输入值_25"(w421) -> ()
        n1304 = local write "输入值_26"(w421) -> ()
        n1305 = local write "输入值_27"(w421) -> ()
        n1306 = local write "输入值_28"(w421) -> ()
        n1307 = local write "输入值_29"(w421) -> ()
        n1308 = local write "输入值_30"(w421) -> ()
        n1309 = local write "输入值_31"(w421) -> ()
        n1310 = local write "输入值_32"(w421) -> ()
        n1311 = local write "输入值_33"(w421) -> ()
        n1312 = local write "输入值_34"(w421) -> ()
        n1313 = local write "输入值_35"(w421) -> ()
        n1314 = local write "输入值_36"(w421) -> ()
        n1315 = local write "输入值_37"(w421) -> ()
        n1316 = local write "输入值_38"(w421) -> ()
        n1317 = local write "输入值_39"(w421) -> ()
        n1318 = local write "输入值_40"(w421) -> ()
        n1319 = local write "输入值_41"(w421) -> ()
        n1320 = local write "输入值_42"(w421) -> ()
        n1321 = local write "输入值_43"(w421) -> ()
        n1322 = local write "输入值_44"(w421) -> ()
        n1323 = local write "输入值_45"(w421) -> ()
        n1324 = local write "输入值_46"(w421) -> ()
        n1325 = local write "输入值_47"(w421) -> ()
        n1326 = local write "输入值_48"(w421) -> ()
        n1327 = local write "输入值_49"(w421) -> ()
        n1328 = local write "输入值_50"(w421) -> ()
        n1329 = local write "输入值_51"(w421) -> ()
        n1330 = local write "输入值_52"(w421) -> ()
        n1331 = local write "输入值_53"(w421) -> ()
        n1332 = local write "输入值_54"(w421) -> ()
        n1333 = local write "输入值_55"(w421) -> ()
        n1334 = local write "输入值_56"(w421) -> ()
        n1335 = local write "输入值_57"(w421) -> ()
        n1336 = local write "输入值_58"(w421) -> ()
        n1337 = local write "输入值_59"(w421) -> ()
        n1338 = local write "输入值_60"(w421) -> ()
        n1339 = local write "输入值_61"(w421) -> ()
        n1340 = local write "输入值_62"(w421) -> ()
        n1341 = local write "输入值_63"(w421) -> ()
        n1342 = local write "输入值_64"(w421) -> ()
        n1343 = local write "输入值_65"(w421) -> ()
        n1344 = local write "输入值_66"(w421) -> ()
        n1345 = local write "输入值_67"(w421) -> ()
        n1346 = local write "输入值_68"(w421) -> ()
        n1347 = local write "输入值_69"(w421) -> ()
        n1348 = local write "输入值_70"(w421) -> ()
        n1349 = local write "输入值_71"(w421) -> ()
        n1350 = local write "输入值_72"(w421) -> ()
        n1351 = local write "输入值_73"(w421) -> ()
        n1352 = local write "输入值_74"(w421) -> ()
        n1353 = local write "输入值_75"(w421) -> ()
        n1354 = local write "输入值_76"(w421) -> ()
        n1355 = local write "输入值_77"(w421) -> ()
        n1356 = local write "输入值_78"(w421) -> ()
        n1357 = local write "输入值_79"(w421) -> ()
        n1358 = local write "输入值_80"(w421) -> ()
      }
    }
  }
  n1359 = stacked-sequence {
    frame #0 {
      w429 = 0 ("同步_A1")
      w441 = T1."Disabled" ("禁用")
      n1360 = property on="测试结论" class="Str"("Text.TextColor"=u32 0) -> ()  [unwired: 2 in, 2 out]
      n1361 = local write "测试结论"("") -> ()
      n1362 = local write "CAN端口"(u16 1 ("CAN端口")) -> ()
      n1363 = local write "同步_A1"(w429) -> ()
      n1364 = local write "同步_A2"(w429) -> ()
      n1365 = property on="D_IN_1" class="Tbl (严格)"("DisabledEnum"=w441) -> ()  [unwired: 2 in, 2 out]
      n1366 = property on="D_IN_2" class="Tbl (严格)"("DisabledEnum"=w441) -> ()  [unwired: 2 in, 2 out]
      n1367 = property on="D_IN_3" class="Tbl (严格)"("DisabledEnum"=w441) -> ()  [unwired: 2 in, 2 out]
      n1368 = property on="D_IN_4" class="Tbl (严格)"("DisabledEnum"=w441) -> ()  [unwired: 2 in, 2 out]
      n1369 = property on="D_IN_5" class="Tbl (严格)"("DisabledEnum"=w441) -> ()  [unwired: 2 in, 2 out]
      n1370 = property on="btn_开始试验" class="Bool"("DisabledEnum"=T1."Enabled" ("禁用")) -> ()  [unwired: 2 in, 2 out]
      n1371 = for {
        N: 16 -> [_]
        i -> [w482]
        n1372 = for {
          N: 4 -> [_]
          tunnel: w482 -> [w486]
          i -> [w487]
          w484 = u32 24 ("活动单元格:单元格大小:高度")
          n1373 = Bundle(w486, w487) -> (w485:cluster{i32, i32})  [unwired: 1 in]
          n1374 = property on="D_IN_1" class="Tbl (严格)"("Active Cell"=w485) -> (error out=w488:errorcluster)  [unwired: 2 in, 1 out]
          n1375 = property on="D_IN_2" class="Tbl (严格)"("Active Cell"=w485) -> ()  [unwired: 2 in, 2 out]
          n1376 = property on="D_IN_3" class="Tbl (严格)"("Active Cell"=w485) -> ()  [unwired: 2 in, 2 out]
          n1377 = property on="D_IN_4" class="Tbl (严格)"("Active Cell"=w485) -> ()  [unwired: 2 in, 2 out]
          n1378 = property on="D_IN_5" class="Tbl (严格)"("Active Cell"=w485) -> ()  [unwired: 2 in, 2 out]
          n1379 = property on="D_IN_1" class="Tbl (严格)"(error in=w488, "Height"=w484) -> ()  [unwired: 1 in, 2 out]
          n1380 = property on="D_IN_2" class="Tbl (严格)"("Height"=w484) -> ()  [unwired: 2 in, 2 out]
          n1381 = property on="D_IN_3" class="Tbl (严格)"("Height"=w484) -> ()  [unwired: 2 in, 2 out]
          n1382 = property on="D_IN_4" class="Tbl (严格)"("Height"=w484) -> ()  [unwired: 2 in, 2 out]
          n1383 = property on="D_IN_5" class="Tbl (严格)"("Height"=w484) -> ()  [unwired: 2 in, 2 out]
        }
        n1384 = Wait Until Next ms Multiple(millisecond multiple=u32 10 ("毫秒倍数")) -> ()  [unwired: 1 out]
      }
      n1385 = Initialize Array(FALSE, 80 ("维数大小")) -> (w425:bool[])
      n1386 = Initialize Array(enum16{"0", "1"}."0" ("输入值_32"), 80 ("维数大小")) -> (w426:enum16{"0", "1"}[])
      n1387 = Initialize Array("", 16 ("维数大小"), 4 ("维数大小")) -> (w435:string[][])
      n1388 = local write "关闭？"(FALSE) -> ()
      n1389 = local write "数组_选择?"(w425) -> ()
      n1390 = local write "数组_输入值"(w426) -> ()
      n1391 = local write "D_IN_1"(w435) -> ()
      n1392 = local write "D_IN_2"(w435) -> ()
      n1393 = local write "D_IN_3"(w435) -> ()
      n1394 = local write "D_IN_4"(w435) -> ()
      n1395 = local write "D_IN_5"(w435) -> ()
      n1396 = Initialize Array(FALSE, 80 ("维数大小")) -> (w422:bool[])
      n1397 = local write "第几组数据"(0 ("第几组数据")) -> ()
      n1398 = local write "合格？"(w422) -> ()
      n1399 = stacked-sequence {
        frame #0 {
          # "初始化配置文件路径"
          n1400 = VI Library "VI库"() -> (path=w449:path)
          n1401 = Strip Path(path=w449) -> (stripped path=w448:path)  [unwired: 1 out]
          n1402 = Build Path(base path=w448, name or relative path="config" ("名称或相对路径")) -> (appended path=w446:path)
          n1403 = Build Path(base path=w446, name or relative path="bordII_config" ("名称或相对路径")) -> (appended path=w444:path)
          n1404 = local write "配置文件目录 2"(w444) -> ()
        }
        frame #1 {
          # "遍历配置文件目录"
          n1405 = local read "配置文件目录 2"() -> (w451:path)
          n1406 = call "罗列目录配置文件.vi"("路径"=w451) -> ("数组"=w450:string[])  [unwired: 10 in]
          n1407 = property on="加载配置文件" class="Ring (严格)"("Strings []"=w450) -> ()  [unwired: 2 in, 2 out]
        }
        frame #2 {
          n1408 = property on="加载配置文件" class="Ring (严格)"() -> ("RingText.Text"=w452:string)  [unwired: 2 in, 2 out]
          n1409 = local write "加载文件名称"(w452) -> ()
        }
        frame #3 {
          # "待读取配置文件路径"
          n1410 = local read "配置文件目录 2"() -> (w454:path)
          n1411 = property on="加载文件名称" class="Str"() -> ("Text.Text"=w453:string)  [unwired: 2 in, 2 out]
          n1412 = Build Path(base path=w454, name or relative path=w453) -> (appended path=w455:path)
          n1413 = local write "配置文件路径"(w455) -> ()
        }
        frame #4 {
          # "读取默认配置的配置内容"
          n1414 = local read "配置文件路径"() -> (w457:path)
          n1415 = call "函数测试配置文件读取.vi"("配置文件路径"=w457) -> ("D_IN_3"=w456:string[][])  [unwired: 6 in, 3 out]
          n1416 = local write "D_IN_1 2"(w456) -> ()
        }
        frame #5 {
          n1417 = for {
            N: 80 -> [_]
            tunnel: [w478] -> w462 mode=indexing
            tunnel: [w475] -> w461 mode=indexing
            tunnel: [w472] -> w460 mode=indexing
            tunnel: [w469] -> w459 mode=indexing
            tunnel: [w464] -> w458 mode=indexing
            i -> [w466]
            n1418 = local read "D_IN_1 2"() -> (w467:string[][])
            n1419 = Index Array(array=w467, index (row)=w466, index (col)=1 ("禁用的索引 (列)")) -> (element=w477:string)
            n1420 = Index Array(array=w467, index (row)=w466, index (col)=3 ("禁用的索引 (列)")) -> (element=w473:string)
            n1421 = Index Array(array=w467, index (row)=w466, index (col)=5 ("禁用的索引 (列)")) -> (element=w465:string)
            n1422 = Index Array(array=w467, index (row)=w466, index (col)=2 ("禁用的索引 (列)")) -> (element=w479:string)
            n1423 = Index Array(array=w467, index (row)=w466, index (col)=4 ("禁用的索引 (列)")) -> (element=w470:string)
            n1424 = Decimal String To Number(string=w477) -> (number=w475:i32)  [unwired: 2 in, 1 out]
            n1425 = Decimal String To Number(string=w473) -> (number=w472:i32)  [unwired: 2 in, 1 out]
            n1426 = Decimal String To Number(string=w465) -> (number=w464:i32)  [unwired: 2 in, 1 out]
            n1427 = Decimal String To Number(string=w479) -> (number=w478:i32)  [unwired: 2 in, 1 out]
            n1428 = Decimal String To Number(string=w470) -> (number=w469:i32)  [unwired: 2 in, 1 out]
          }
          n1429 = global write "试验配置信息.vi" "设定输出通道"(w461) -> ()
          n1430 = global write "试验配置信息.vi" "输出切换ID"(w460) -> ()
          n1431 = global write "试验配置信息.vi" "跳变方向"(w458) -> ()
          n1432 = global write "试验配置信息.vi" "设定输入通道"(w462) -> ()
          n1433 = global write "试验配置信息.vi" "输入切换ID"(w459) -> ()
        }
      }
    }
  }
  n1434 = Obtain Notifier(name (unnamed)=w2, notification data type=w2) -> (notifier out=w10:refnum<notifier>, error out=w9:errorcluster)  [unwired: 2 in, 1 out]
  n1435 = while {
    tunnel: w10 -> [w493]
    tunnel: w9 -> [w492]
    tunnel: [w491] -> w8
    tunnel: [w490] -> w7
    stop <- w494 stop-if-true
    n1436 = Wait Until Next ms Multiple(millisecond multiple=u32 20 ("毫秒倍数")) -> ()  [unwired: 1 out]
    n1437 = Wait on Notification(notifier=w493, timeout in ms (-1)=20 ("超时毫秒(-1)"), error in (no error)=w492) -> (notifier out=w491:refnum<notifier>, notification=w498:string, error out=w490:errorcluster)  [unwired: 1 in, 1 out]
    n1438 = Equal?(x=w498, y="DInput" ("通知")) -> (x = y?=w489:bool)
    n1439 = case shown="真" w489 {
      frame False {
      }
      frame True {
        n1440 = stacked-sequence {
          frame #0 {
            n1441 = for {
              N: 80 -> [_]
              i -> [w501]
              n1442 = local read "数组_选择?"() -> (w503:bool[])
              n1443 = local read "数组_输入值"() -> (w500:enum16{"0", "1"}[])
              n1444 = Index Array(array=w503, index=w501) -> (element=w502:bool)
              n1445 = case shown="真" w502 {
                tunnel: w501 -> [_ w507]
                tunnel: w501 -> [_ w505]
                tunnel: w500 -> [_ w504]
                frame False {
                }
                frame True {
                  n1446 = local read "CAN端口"() -> (w509:u16)
                  n1447 = Increment(x=w507) -> (x+1=w508:i32)
                  n1448 = call "16路数字量输入.vi"("第几组数据"=w508, "CAN端口"=w509) -> ()  [unwired: 9 in, 1 out]
                  n1449 = case shown="真" TRUE {
                    tunnel: w505 -> [_ w511]
                    tunnel: w504 -> [_ w510]
                    frame False {
                    }
                    frame True {
                      n1450 = while {
                        tunnel: w511 -> [w516]
                        tunnel: w510 -> [w515]
                        stop <- w514 stop-if-true
                        n1451 = local read "同步_A1"() -> (w512:i32)
                        n1452 = Wait Until Next ms Multiple(millisecond multiple=u32 10 ("毫秒倍数")) -> ()  [unwired: 1 out]
                        n1453 = Equal?(x=w512, y=0) -> (x = y?=w517:bool)
                        n1454 = case shown="真" w517 {
                          tunnel: w516 -> [_ w522]
                          tunnel: w515 -> [_ w521]
                          tunnel: [FALSE w520] -> w514
                          frame False {
                          }
                          frame True {
                            n1455 = stacked-sequence {
                              tunnel: w522 -> [_ w534 _ _]
                              tunnel: w521 -> [_ w533 _ _]
                              tunnel: [_ _ _ w593] -> w520
                              frame #0 {
                                n1456 = Wait (ms)(milliseconds to wait=u32 100) -> ()  [unwired: 1 out]
                              }
                              frame #1 {
                                n1457 = To Long Integer(number=w534) -> (32bit integer=w524:i32)
                                n1458 = global read "试验配置信息.vi" "设定输出通道"() -> (w535:i32[])
                                n1459 = Index Array(array=w533, index=w524) -> (element=w531:enum16{"0", "1"})
                                n1460 = local write "第几组数据"(w524) -> ()
                                n1461 = Index Array(array=w535, index=w524) -> (element=w532:i32)
                                n1462 = case shown="0, 默认" w532 {
                                tunnel: w531 -> [w542 w545 w547 w550 w553 w556 w559 w562 w565 w568 w571 w574 w577 w580 w583 w586]
                                tunnel: [w541 w544 w548 w551 w554 w557 w560 w563 w566 w569 w572 w575 w578 w581 w584 w587] -> w525
                                frame 0, Default {
                                w540 = 0 ("y")
                                n1463 = Build Array(w542, w540, w540, w540, w540, w540, w540, w540, w540, w540, w540, w540, w540, w540, w540, w540) -> (w541:i32[])
                                }
                                frame 1 {
                                w543 = 0 ("y")
                                n1464 = Build Array(w543, w545, w543, w543, w543, w543, w543, w543, w543, w543, w543, w543, w543, w543, w543, w543) -> (w544:i32[])
                                }
                                frame 2 {
                                w546 = 0 ("y")
                                n1465 = Build Array(w546, w546, w547, w546, w546, w546, w546, w546, w546, w546, w546, w546, w546, w546, w546, w546) -> (w548:i32[])
                                }
                                frame 3 {
                                w549 = 0 ("y")
                                n1466 = Build Array(w549, w549, w549, w550, w549, w549, w549, w549, w549, w549, w549, w549, w549, w549, w549, w549) -> (w551:i32[])
                                }
                                frame 4 {
                                w552 = 0 ("y")
                                n1467 = Build Array(w552, w552, w552, w552, w553, w552, w552, w552, w552, w552, w552, w552, w552, w552, w552, w552) -> (w554:i32[])
                                }
                                frame 5 {
                                w555 = 0 ("y")
                                n1468 = Build Array(w555, w555, w555, w555, w555, w556, w555, w555, w555, w555, w555, w555, w555, w555, w555, w555) -> (w557:i32[])
                                }
                                frame 6 {
                                w558 = 0 ("y")
                                n1469 = Build Array(w558, w558, w558, w558, w558, w558, w559, w558, w558, w558, w558, w558, w558, w558, w558, w558) -> (w560:i32[])
                                }
                                frame 7 {
                                w561 = 0 ("y")
                                n1470 = Build Array(w561, w561, w561, w561, w561, w561, w561, w562, w561, w561, w561, w561, w561, w561, w561, w561) -> (w563:i32[])
                                }
                                frame 8 {
                                w564 = 0 ("y")
                                n1471 = Build Array(w564, w564, w564, w564, w564, w564, w564, w564, w565, w564, w564, w564, w564, w564, w564, w564) -> (w566:i32[])
                                }
                                frame 9 {
                                w567 = 0 ("y")
                                n1472 = Build Array(w567, w567, w567, w567, w567, w567, w567, w567, w567, w568, w567, w567, w567, w567, w567, w567) -> (w569:i32[])
                                }
                                frame 10 {
                                w570 = 0 ("y")
                                n1473 = Build Array(w570, w570, w570, w570, w570, w570, w570, w570, w570, w570, w571, w570, w570, w570, w570, w570) -> (w572:i32[])
                                }
                                frame 11 {
                                w573 = 0 ("y")
                                n1474 = Build Array(w573, w573, w573, w573, w573, w573, w573, w573, w573, w573, w573, w574, w573, w573, w573, w573) -> (w575:i32[])
                                }
                                frame 12 {
                                w576 = 0 ("y")
                                n1475 = Build Array(w576, w576, w576, w576, w576, w576, w576, w576, w576, w576, w576, w576, w577, w576, w576, w576) -> (w578:i32[])
                                }
                                frame 13 {
                                w579 = 0 ("y")
                                n1476 = Build Array(w579, w579, w579, w579, w579, w579, w579, w579, w579, w579, w579, w579, w579, w580, w579, w579) -> (w581:i32[])
                                }
                                frame 14 {
                                w582 = 0 ("y")
                                n1477 = Build Array(w582, w582, w582, w582, w582, w582, w582, w582, w582, w582, w582, w582, w582, w582, w583, w582) -> (w584:i32[])
                                }
                                frame 15 {
                                w585 = 0 ("y")
                                n1478 = Build Array(w585, w585, w585, w585, w585, w585, w585, w585, w585, w585, w585, w585, w585, w585, w585, w586) -> (w587:i32[])
                                }
                                }
                                n1479 = for {
                                tunnel: w525 -> [w537] mode=indexing
                                tunnel: [w536] -> w530 mode=indexing
                                n1480 = case shown="1" w537 {
                                tunnel: [FALSE TRUE] -> w536
                                frame 0, Default {
                                }
                                frame 1 {
                                }
                                }
                                }
                                n1481 = Boolean Array To Number ("布尔数组至数值转换")(Boolean array=w530) -> (number=w529:u16)
                                n1482 = Split Number(x=w529) -> (hi(x)=w526:u8, lo(x)=w527:u8)
                                n1483 = Build Array(w527, w526) -> (w528:u8[])
                                n1484 = call "DO"("dataIn(U8Array)"=w528) -> ()  [unwired: 2 in, 17 out]
                              }
                              frame #2 {
                                w592 = "DICheckStart" ("名称（未命名）")
                                n1485 = local write "同步_A1"(1 ("同步_A1")) -> ()
                                n1486 = Obtain Notifier(name (unnamed)=w592, notification data type=w592) -> (notifier out=w591:refnum<notifier>, error out=w590:errorcluster)  [unwired: 2 in, 1 out]
                                n1487 = Send Notification(notification="DICheck" ("通知"), notifier=w591, error in (no error)=w590) -> ()  [unwired: 2 out]
                              }
                              frame #3 {
                                n1488 = local read "同步_A1"() -> (w594:i32)
                                n1489 = Equal?(x=w594, y=1) -> (x = y?=w593:bool)
                              }
                            }
                          }
                        }
                      }
                    }
                  }
                }
              }
            }
          }
          frame #1 {
            n1490 = property on="btn_关闭" class="Bool"("DisabledEnum"=T1."Enabled" ("禁用")) -> ()  [unwired: 2 in, 2 out]
          }
        }
      }
    }
    n1491 = local read "关闭？"() -> (w494:bool)
  }
  n1492 = Release Notifier(notifier=w8, error in (no error)=w7) -> ()  [unwired: 1 in, 3 out]
  n1493 = disable-structure shown="启用" {
    frame Disabled {
      n1494 = for {
        N: 40 -> [_]
        i -> [w602]
        n1495 = Wait Until Next ms Multiple(millisecond multiple=u32 10 ("毫秒倍数")) -> ()  [unwired: 1 out]
        n1496 = Bundle(w602, "y"=-1) -> (w601:cluster{i32, "y":i32})  [unwired: 1 in]
        n1497 = property on="D_IN_1" class="Tbl (严格)"("Active Cell"=w601) -> (error out=w600:errorcluster)  [unwired: 2 in, 1 out]
        n1498 = property on="D_IN_1" class="Tbl (严格)"(error in=w600, "Cell BG Color"=u32 12369084) -> ()  [unwired: 1 in, 2 out]
      }
    }
    frame Enabled {
    }
  }
  n1499 = disable-structure shown="启用" {
    frame Disabled {
      n1500 = for {
        N: 40 -> [_]
        i -> [w606]
        n1501 = for {
          N: 4 -> [_]
          tunnel: w606 -> [w614]
          i -> [w611]
          n1502 = Bundle(w614, w611) -> (w610:cluster{i32, i32})  [unwired: 1 in]
          n1503 = Quotient & Remainder(x=w614, y=2) -> (x-y*floor(x/y)=w612:i32)  [unwired: 1 out]
          n1504 = property on="D_IN_1" class="Tbl (严格)"("Active Cell"=w610) -> (error out=w608:errorcluster)  [unwired: 2 in, 1 out]
          n1505 = Equal To 0?(x=w612) -> (x = 0?=w615:bool)
          n1506 = case shown="真" w615 {
            tunnel: [u32 16448250 u32 15723488] -> w609
            frame False {
            }
            frame True {
            }
          }
          n1507 = property on="D_IN_1" class="Tbl (严格)"(error in=w608, "Cell BG Color"=w609) -> ()  [unwired: 1 in, 2 out]
        }
        n1508 = Wait Until Next ms Multiple(millisecond multiple=u32 10 ("毫秒倍数")) -> ()  [unwired: 1 out]
      }
    }
    frame Enabled {
    }
  }
  n1509 = Obtain Notifier(name (unnamed)=w1, notification data type=w1) -> (notifier out=w6:refnum<notifier>, error out=w5:errorcluster)  [unwired: 2 in, 1 out]
  n1510 = while {
    tunnel: w6 -> [w622]
    tunnel: w5 -> [w621]
    tunnel: [w620] -> w4
    tunnel: [w619] -> w3
    stop <- w624 stop-if-true
    n1511 = Wait Until Next ms Multiple(millisecond multiple=u32 20 ("毫秒倍数")) -> ()  [unwired: 1 out]
    n1512 = Wait on Notification(notifier=w622, timeout in ms (-1)=20 ("超时毫秒(-1)"), error in (no error)=w621) -> (notifier out=w620:refnum<notifier>, notification=w625:string, error out=w619:errorcluster)  [unwired: 1 in, 1 out]
    n1513 = Equal?(x=w625, y="DICheck" ("通知")) -> (x = y?=w623:bool)
    n1514 = case shown="真" w623 {
      frame False {
      }
      frame True {
        n1515 = stacked-sequence {
          frame #0 {
            n1516 = local read "数组_输入值"() -> (w645:enum16{"0", "1"}[])
            n1517 = local read "第几组数据"() -> (w642:i32)
            n1518 = global read "试验配置信息.vi" "跳变方向"() -> (w647:i32[])
            n1519 = global read "试验配置信息.vi" "设定输入通道"() -> (w656:i32[])
            n1520 = Index Array(array=w645, index=w642) -> (element=w644:enum16{"0", "1"})
            n1521 = Index Array(array=w656, index=w642) -> (element=w629:i32)
            n1522 = Index Array(array=w647, index=w642) -> (element=w648:i32)
            n1523 = To Word Integer ("转换为双字节整型")(number=w644) -> (16bit integer=w646:i16)
            n1524 = call "DAQNavi Assistant"() -> ("dataOut(U8Array)"=w655:u8[])  [unwired: 2 in, 17 out]
            n1525 = Equal To 0?(x=w648) -> (x = 0?=w649:bool)
            n1526 = Not Equal To 0?(x=w646) -> (x != 0?=w650:bool)
            n1527 = Index Array(array=w655, index #1=0 ("索引"), index #2=1 ("索引")) -> (element #1=w633:u8, element #2=w632:u8)
            n1528 = case shown="真" w649 {
              tunnel: w650 -> [w770 w771]
              tunnel: [w769 w771] -> w651
              frame False {
                n1529 = Not(x=w770) -> (.not. x?=w769:bool)
              }
              frame True {
              }
            }
            n1530 = Number To Boolean Array(number=w633) -> (Boolean array=w637:bool[])
            n1531 = Number To Boolean Array(number=w632) -> (Boolean array=w636:bool[])
            n1532 = Build Array (concatenate)(w637, w636) -> (w631:bool[])
            n1533 = Boolean To (0,1)(Boolean=w651) -> (0, 1=w652:i16)
            n1534 = Boolean To (0,1) ("布尔值至(0,1)转换")(Boolean=w631) -> (0, 1=w630:i16[])
            n1535 = Index Array(array=w630, index=w629) -> (element=w628:i16)
            n1536 = Equal?(x=w628, y=w652) -> (x = y?=w653:bool)
            n1537 = Equal To 0?(x=w628) -> (x = 0?=w654:bool)
            n1538 = case shown="真" w654 {
              tunnel: ["1" "0"] -> w643
              frame False {
              }
              frame True {
              }
            }
            n1539 = case shown="假" w653 {
              tunnel: [cluster{u32, u32}[] [{16711680, 16711680}] ("结果") cluster{u32, u32}[] [{6618880, 6618880}] ("结果")] -> w638
              frame False {
              }
              frame True {
              }
            }
            n1540 = Quotient & Remainder(x=w642, y=16) -> (x-y*floor(x/y)=w639:i32, floor(x/y)=w640:i32)
            n1541 = case shown="0, 默认" w640 {
              tunnel: w638 -> [w657 w679 w701 w723 w745]
              tunnel: w643 -> [w659 w682 w704 w725 w747]
              tunnel: w639 -> [w658 w680 w702 w724 w746]
              frame 0, Default {
                n1542 = local read "D_IN_1"() -> (w662:string[][])
                n1543 = Replace Array Subset(array=w662, new element=w659, index (row)=w658, index (col)=2 ("禁用的索引 (列)")) -> (w660:string[][])
                n1544 = case shown="15" w658 {
                  tunnel: w657 -> [w663 w664 w665 w666 w667 w668 w669 w670 w671 w672 w673 w674 w675 w676 w677 w678]
                  frame 0, Default {
                    n1545 = property on="light_1" class="Bool (严格)"("Colors [4]"=w663) -> ()  [unwired: 2 in, 2 out]
                  }
                  frame 1 {
                    n1546 = property on="light_2" class="Bool (严格)"("Colors [4]"=w664) -> ()  [unwired: 2 in, 2 out]
                  }
                  frame 3 {
                    n1547 = property on="light_4" class="Bool (严格)"("Colors [4]"=w665) -> ()  [unwired: 2 in, 2 out]
                  }
                  frame 4 {
                    n1548 = property on="light_5" class="Bool (严格)"("Colors [4]"=w666) -> ()  [unwired: 2 in, 2 out]
                  }
                  frame 5 {
                    n1549 = property on="light_6" class="Bool (严格)"("Colors [4]"=w667) -> ()  [unwired: 2 in, 2 out]
                  }
                  frame 6 {
                    n1550 = property on="light_7" class="Bool (严格)"("Colors [4]"=w668) -> ()  [unwired: 2 in, 2 out]
                  }
                  frame 7 {
                    n1551 = property on="light_8" class="Bool (严格)"("Colors [4]"=w669) -> ()  [unwired: 2 in, 2 out]
                  }
                  frame 8 {
                    n1552 = property on="light_9" class="Bool (严格)"("Colors [4]"=w670) -> ()  [unwired: 2 in, 2 out]
                  }
                  frame 9 {
                    n1553 = property on="light_10" class="Bool (严格)"("Colors [4]"=w671) -> ()  [unwired: 2 in, 2 out]
                  }
                  frame 10 {
                    n1554 = property on="light_11" class="Bool (严格)"("Colors [4]"=w672) -> ()  [unwired: 2 in, 2 out]
                  }
                  frame 11 {
                    n1555 = property on="light_12" class="Bool (严格)"("Colors [4]"=w673) -> ()  [unwired: 2 in, 2 out]
                  }
                  frame 12 {
                    n1556 = property on="light_13" class="Bool (严格)"("Colors [4]"=w674) -> ()  [unwired: 2 in, 2 out]
                  }
                  frame 13 {
                    n1557 = property on="light_14" class="Bool (严格)"("Colors [4]"=w675) -> ()  [unwired: 2 in, 2 out]
                  }
                  frame 14 {
                    n1558 = property on="light_15" class="Bool (严格)"("Colors [4]"=w676) -> ()  [unwired: 2 in, 2 out]
                  }
                  frame 15 {
                    n1559 = property on="light_16" class="Bool (严格)"("Colors [4]"=w677) -> ()  [unwired: 2 in, 2 out]
                  }
                  frame 2 {
                    n1560 = property on="light_3" class="Bool (严格)"("Colors [4]"=w678) -> ()  [unwired: 2 in, 2 out]
                  }
                }
                n1561 = local write "D_IN_1"(w660) -> ()
              }
              frame 2 {
                n1562 = local read "D_IN_3"() -> (w683:string[][])
                n1563 = case shown="15" w680 {
                  tunnel: w679 -> [w685 w686 w687 w688 w689 w690 w691 w692 w693 w694 w695 w696 w697 w698 w699 w700]
                  frame 0, Default {
                    n1564 = property on="light_33" class="Bool (严格)"("Colors [4]"=w685) -> ()  [unwired: 2 in, 2 out]
                  }
                  frame 1 {
                    n1565 = property on="light_34" class="Bool (严格)"("Colors [4]"=w686) -> ()  [unwired: 2 in, 2 out]
                  }
                  frame 2 {
                    n1566 = property on="light_35" class="Bool (严格)"("Colors [4]"=w687) -> ()  [unwired: 2 in, 2 out]
                  }
                  frame 3 {
                    n1567 = property on="light_36" class="Bool (严格)"("Colors [4]"=w688) -> ()  [unwired: 2 in, 2 out]
                  }
                  frame 4 {
                    n1568 = property on="light_37" class="Bool (严格)"("Colors [4]"=w689) -> ()  [unwired: 2 in, 2 out]
                  }
                  frame 5 {
                    n1569 = property on="light_38" class="Bool (严格)"("Colors [4]"=w690) -> ()  [unwired: 2 in, 2 out]
                  }
                  frame 6 {
                    n1570 = property on="light_39" class="Bool (严格)"("Colors [4]"=w691) -> ()  [unwired: 2 in, 2 out]
                  }
                  frame 7 {
                    n1571 = property on="light_40" class="Bool (严格)"("Colors [4]"=w692) -> ()  [unwired: 2 in, 2 out]
                  }
                  frame 8 {
                    n1572 = property on="light_41" class="Bool (严格)"("Colors [4]"=w693) -> ()  [unwired: 2 in, 2 out]
                  }
                  frame 9 {
                    n1573 = property on="light_42" class="Bool (严格)"("Colors [4]"=w694) -> ()  [unwired: 2 in, 2 out]
                  }
                  frame 10 {
                    n1574 = property on="light_43" class="Bool (严格)"("Colors [4]"=w695) -> ()  [unwired: 2 in, 2 out]
                  }
                  frame 11 {
                    n1575 = property on="light_44" class="Bool (严格)"("Colors [4]"=w696) -> ()  [unwired: 2 in, 2 out]
                  }
                  frame 12 {
                    n1576 = property on="light_45" class="Bool (严格)"("Colors [4]"=w697) -> ()  [unwired: 2 in, 2 out]
                  }
                  frame 13 {
                    n1577 = property on="light_46" class="Bool (严格)"("Colors [4]"=w698) -> ()  [unwired: 2 in, 2 out]
                  }
                  frame 14 {
                    n1578 = property on="light_47" class="Bool (严格)"("Colors [4]"=w699) -> ()  [unwired: 2 in, 2 out]
                  }
                  frame 15 {
                    n1579 = property on="light_48" class="Bool (严格)"("Colors [4]"=w700) -> ()  [unwired: 2 in, 2 out]
                  }
                }
                n1580 = Replace Array Subset(array=w683, new element=w682, index (row)=w680, index (col)=2 ("索引 (列)")) -> (w681:string[][])
                n1581 = local write "D_IN_3"(w681) -> ()
              }
              frame 3 {
                n1582 = local read "D_IN_4"() -> (w705:string[][])
                n1583 = case shown="15" w702 {
                  tunnel: w701 -> [w707 w708 w709 w710 w711 w712 w713 w714 w715 w716 w717 w718 w719 w720 w721 w722]
                  frame 0, Default {
                    n1584 = property on="light_49" class="Bool (严格)"("Colors [4]"=w707) -> ()  [unwired: 2 in, 2 out]
                  }
                  frame 1 {
                    n1585 = property on="light_50" class="Bool (严格)"("Colors [4]"=w708) -> ()  [unwired: 2 in, 2 out]
                  }
                  frame 2 {
                    n1586 = property on="light_51" class="Bool (严格)"("Colors [4]"=w709) -> ()  [unwired: 2 in, 2 out]
                  }
                  frame 3 {
                    n1587 = property on="light_52" class="Bool (严格)"("Colors [4]"=w710) -> ()  [unwired: 2 in, 2 out]
                  }
                  frame 4 {
                    n1588 = property on="light_53" class="Bool (严格)"("Colors [4]"=w711) -> ()  [unwired: 2 in, 2 out]
                  }
                  frame 5 {
                    n1589 = property on="light_54" class="Bool (严格)"("Colors [4]"=w712) -> ()  [unwired: 2 in, 2 out]
                  }
                  frame 6 {
                    n1590 = property on="light_55" class="Bool (严格)"("Colors [4]"=w713) -> ()  [unwired: 2 in, 2 out]
                  }
                  frame 7 {
                    n1591 = property on="light_56" class="Bool (严格)"("Colors [4]"=w714) -> ()  [unwired: 2 in, 2 out]
                  }
                  frame 8 {
                    n1592 = property on="light_57" class="Bool (严格)"("Colors [4]"=w715) -> ()  [unwired: 2 in, 2 out]
                  }
                  frame 9 {
                    n1593 = property on="light_58" class="Bool (严格)"("Colors [4]"=w716) -> ()  [unwired: 2 in, 2 out]
                  }
                  frame 10 {
                    n1594 = property on="light_59" class="Bool (严格)"("Colors [4]"=w717) -> ()  [unwired: 2 in, 2 out]
                  }
                  frame 11 {
                    n1595 = property on="light_60" class="Bool (严格)"("Colors [4]"=w718) -> ()  [unwired: 2 in, 2 out]
                  }
                  frame 12 {
                    n1596 = property on="light_61" class="Bool (严格)"("Colors [4]"=w719) -> ()  [unwired: 2 in, 2 out]
                  }
                  frame 13 {
                    n1597 = property on="light_62" class="Bool (严格)"("Colors [4]"=w720) -> ()  [unwired: 2 in, 2 out]
                  }
                  frame 14 {
                    n1598 = property on="light_63" class="Bool (严格)"("Colors [4]"=w721) -> ()  [unwired: 2 in, 2 out]
                  }
                  frame 15 {
                    n1599 = property on="light_64" class="Bool (严格)"("Colors [4]"=w722) -> ()  [unwired: 2 in, 2 out]
                  }
                }
                n1600 = Replace Array Subset(array=w705, new element=w704, index (row)=w702, index (col)=2 ("索引 (列)")) -> (w703:string[][])
                n1601 = local write "D_IN_4"(w703) -> ()
              }
              frame 4 {
                n1602 = local read "D_IN_5"() -> (w727:string[][])
                n1603 = case shown="15" w724 {
                  tunnel: w723 -> [w729 w730 w731 w732 w733 w734 w735 w736 w737 w738 w739 w740 w741 w742 w743 w744]
                  frame 0, Default {
                    n1604 = property on="light_65" class="Bool (严格)"("Colors [4]"=w729) -> ()  [unwired: 2 in, 2 out]
                  }
                  frame 1 {
                    n1605 = property on="light_66" class="Bool (严格)"("Colors [4]"=w730) -> ()  [unwired: 2 in, 2 out]
                  }
                  frame 2 {
                    n1606 = property on="light_67" class="Bool (严格)"("Colors [4]"=w731) -> ()  [unwired: 2 in, 2 out]
                  }
                  frame 3 {
                    n1607 = property on="light_68" class="Bool (严格)"("Colors [4]"=w732) -> ()  [unwired: 2 in, 2 out]
                  }
                  frame 4 {
                    n1608 = property on="light_69" class="Bool (严格)"("Colors [4]"=w733) -> ()  [unwired: 2 in, 2 out]
                  }
                  frame 5 {
                    n1609 = property on="light_70" class="Bool (严格)"("Colors [4]"=w734) -> ()  [unwired: 2 in, 2 out]
                  }
                  frame 6 {
                    n1610 = property on="light_71" class="Bool (严格)"("Colors [4]"=w735) -> ()  [unwired: 2 in, 2 out]
                  }
                  frame 7 {
                    n1611 = property on="light_72" class="Bool (严格)"("Colors [4]"=w736) -> ()  [unwired: 2 in, 2 out]
                  }
                  frame 8 {
                    n1612 = property on="light_73" class="Bool (严格)"("Colors [4]"=w737) -> ()  [unwired: 2 in, 2 out]
                  }
                  frame 9 {
                    n1613 = property on="light_74" class="Bool (严格)"("Colors [4]"=w738) -> ()  [unwired: 2 in, 2 out]
                  }
                  frame 10 {
                    n1614 = property on="light_75" class="Bool (严格)"("Colors [4]"=w739) -> ()  [unwired: 2 in, 2 out]
                  }
                  frame 11 {
                    n1615 = property on="light_76" class="Bool (严格)"("Colors [4]"=w740) -> ()  [unwired: 2 in, 2 out]
                  }
                  frame 12 {
                    n1616 = property on="light_77" class="Bool (严格)"("Colors [4]"=w741) -> ()  [unwired: 2 in, 2 out]
                  }
                  frame 13 {
                    n1617 = property on="light_78" class="Bool (严格)"("Colors [4]"=w742) -> ()  [unwired: 2 in, 2 out]
                  }
                  frame 14 {
                    n1618 = property on="light_79" class="Bool (严格)"("Colors [4]"=w743) -> ()  [unwired: 2 in, 2 out]
                  }
                  frame 15 {
                    n1619 = property on="light_80" class="Bool (严格)"("Colors [4]"=w744) -> ()  [unwired: 2 in, 2 out]
                  }
                }
                n1620 = Replace Array Subset(array=w727, new element=w725, index (row)=w724, index (col)=2 ("索引 (列)")) -> (w726:string[][])
                n1621 = local write "D_IN_5"(w726) -> ()
              }
              frame 1 {
                n1622 = local read "D_IN_2"() -> (w749:string[][])
                n1623 = case shown="15" w746 {
                  tunnel: w745 -> [w751 w752 w753 w754 w755 w756 w757 w758 w759 w760 w761 w762 w763 w764 w765 w766]
                  frame 0, Default {
                    n1624 = property on="light_17" class="Bool (严格)"("Colors [4]"=w751) -> ()  [unwired: 2 in, 2 out]
                  }
                  frame 1 {
                    n1625 = property on="light_18" class="Bool (严格)"("Colors [4]"=w752) -> ()  [unwired: 2 in, 2 out]
                  }
                  frame 2 {
                    n1626 = property on="light_19" class="Bool (严格)"("Colors [4]"=w753) -> ()  [unwired: 2 in, 2 out]
                  }
                  frame 3 {
                    n1627 = property on="light_20" class="Bool (严格)"("Colors [4]"=w754) -> ()  [unwired: 2 in, 2 out]
                  }
                  frame 4 {
                    n1628 = property on="light_21" class="Bool (严格)"("Colors [4]"=w755) -> ()  [unwired: 2 in, 2 out]
                  }
                  frame 5 {
                    n1629 = property on="light_22" class="Bool (严格)"("Colors [4]"=w756) -> ()  [unwired: 2 in, 2 out]
                  }
                  frame 6 {
                    n1630 = property on="light_23" class="Bool (严格)"("Colors [4]"=w757) -> ()  [unwired: 2 in, 2 out]
                  }
                  frame 7 {
                    n1631 = property on="light_24" class="Bool (严格)"("Colors [4]"=w758) -> ()  [unwired: 2 in, 2 out]
                  }
                  frame 8 {
                    n1632 = property on="light_25" class="Bool (严格)"("Colors [4]"=w759) -> ()  [unwired: 2 in, 2 out]
                  }
                  frame 9 {
                    n1633 = property on="light_26" class="Bool (严格)"("Colors [4]"=w760) -> ()  [unwired: 2 in, 2 out]
                  }
                  frame 10 {
                    n1634 = property on="light_27" class="Bool (严格)"("Colors [4]"=w761) -> ()  [unwired: 2 in, 2 out]
                  }
                  frame 11 {
                    n1635 = property on="light_28" class="Bool (严格)"("Colors [4]"=w762) -> ()  [unwired: 2 in, 2 out]
                  }
                  frame 12 {
                    n1636 = property on="light_29" class="Bool (严格)"("Colors [4]"=w763) -> ()  [unwired: 2 in, 2 out]
                  }
                  frame 13 {
                    n1637 = property on="light_30" class="Bool (严格)"("Colors [4]"=w764) -> ()  [unwired: 2 in, 2 out]
                  }
                  frame 14 {
                    n1638 = property on="light_31" class="Bool (严格)"("Colors [4]"=w765) -> ()  [unwired: 2 in, 2 out]
                  }
                  frame 15 {
                    n1639 = property on="light_32" class="Bool (严格)"("Colors [4]"=w766) -> ()  [unwired: 2 in, 2 out]
                  }
                }
                n1640 = Replace Array Subset(array=w749, new element=w747, index (row)=w746, index (col)=2 ("索引 (列)")) -> (w748:string[][])
                n1641 = local write "D_IN_2"(w748) -> ()
              }
            }
          }
          frame #1 {
            n1642 = local write "同步_A1"(0 ("同步_A1")) -> ()
          }
        }
      }
    }
    n1643 = local read "关闭？"() -> (w624:bool)
  }
  n1644 = Release Notifier(notifier=w4, error in (no error)=w3) -> ()  [unwired: 1 in, 3 out]
